vi "AlliGator Image Actions.vi"(0 "AlliGator Q Elements":T4[](array[typedef]), 1 "VI in":refnum<vi>, 2 "Script in":bool, 5 "AlliGator IV DVR in":refnum<data-value>, 7 "AlliGator Q Event in":T5=enum."GUI:Idle", 9 "Data":variant, 11 "error in (no error)":errorcluster, 12 "AlliGator Ctrl Refnums":T6) -> (3 "Script out":bool, 4 "Alligator Queue Elements":T4[](array[typedef]), 6 "AlliGator IV DVR out":refnum<data-value>, 10 "[Notebook Message]":T1[](array[typedef]) {"Message Style"."Text Alignment" items=["Left", "Right", "Center"]}, 15 "error out":errorcluster)   [LabVIEW 2021, in "AlliGator Action Engine.lvlib"]
doc: "Processes AlliGator source image-related actions."
uses:
  AlliGator Action Engine.lvlib
  AlliGator Internal Variables v2.ctl
  <vilib>/vision/Image Controls.llb/IMAQ Image.ctl
  AlliGator Gate Image Set.ctl
  AlliGator FLI Dataset Type.ctl
  AlliGator Data Series Type.ctl
  AlliGator Dataset Channel.ctl
  AlliGator Gate Arithmetic.ctl
  AlliGator Displayed Image.ctl
  Image/Named ROI Description.ctl
  AlliGator Decay Metadata v3.ctl
  AlliGator Decay Background Subtraction Info.ctl
  AlliGator Baseline Subtraction Method.ctl
  Graphs/XY Graph/XY Graph Plot Shift Parameters.ctl
  Graphs/XY Graph/XY Graph Plot Shift Method.ctl
  AlliGator Decay Extrapolation Parameters.ctl
  Phasor/Calibration Phasor (m, phi).ctl
  Phasor/Phasor Reference Series.ctl
  Phasor/Phasor Calibration Map v2.ctl
  Phasor/Phasor (g, s).ctl
  AlliGator Raw Phasor Plot Data v4.ctl
  Phasor/Phasor Standard Deviation Options.ctl
  AlliGator Phasor Multi-Harmonic Data.ctl
  Phasor/Phasor Harmonic Data.ctl
  AlliGator Decay Fit Options & Parameters v2.ctl
  Fits/IRF(X)PSED/Decay Fit Options v2.ctl
  Fits/Decay Convolution/Decay Model.ctl
  Fits/Residual Type.ctl
  Fits/IRF(X)PSED/Fit Weights Type.ctl
  Fits/Non-linear Fitting Method v2.ctl
  Fits/Fit Calculation Method.ctl
  Fits/Non-linear Fitting Algorithm.ctl
  AlliGator Decay Fit Parameter Constraints 2.ctl
  Fits/IRF(X)PSED/Decay Fit Parameters In List.ctl
  Fits/IRF(X)PSED/MLE Baseline Offset Type.ctl
  AlliGator Decay Preprocessing Parameters.ctl
  Fits/IRF(X)PSED/Decay Fit Parameters & Derived Quantities List.ctl
  AlliGator Parameter Maps Data.ctl
  AlliGator Q Event.ctl
  AlliGator Ctrl Refnums.ctl
  AlliGator Other Ctrl Refnums.ctl
  AlliGator State Indicator.ctl
  AlliGator Main Window Tabs.ctl
  AlliGator Phasor Plot Ctrl Refnums.ctl
  AlliGator Phasor Graph Ctrl Refnums.ctl
  Phasor/Phasor Calibration Type.ctl
  AlliGator Dataset Ctrl Refnums.ctl
  AlliGator Registered Events Ctrl Refnums.ctl
  AlliGator Image Histogram Control Refnums.ctl
  Histograms/Linear Histogram Options.ctl
  Histograms/Histogram Bin Option.ctl
  Histograms/Histogram Bin Position.ctl
  AlliGator Decay Fit Map Control Refnums.ctl
  AlliGator Q Element.ctl
  Notebook/Notebook Message Object.ctl
  Rich Text Box/Text Formatting.ctl
  Rich Text Box/Text Colors.ctl
  Alligator Elements Order in Action Stack.ctl
  AlliGator Variables List.ctl
  Palette/Image Palette Information.ctl
  Image/Image Display Palette Type.ctl
  Image/Image Display to Clipboard Options.ctl
  AlliGator Settings List.ctl
  AlliGator ROI Manager Actions.ctl
  Image/Image Control ROI Description.ctl
  Image/Image Save File Format.ctl
  AlliGator Saved TIFF Image Type.ctl
  AlliGator Selected ROI.ctl
  Image/Image Control Refnum.ctl
  Utilities/Read-Write.ctl
  5e39216f-2ed3-4ea3-88fe-69bdc2580e7f.vi
  Variant/Variant to Data/Variant to [String].vi
  Variant/Variant to Data/Variant to String.vi
  AlliGator Add Single Action to Stack.vi
  Variant/Variant to Data/Variant to Boolean.vi
  Variant/Variant to Data/Variant to DBL.vi
  AlliGator Source Image ROI Storage [SGL] v3.vi
  AlliGator Add Action Array to Stack.vi
  Variant/Variant to Data/Variant to I32.vi
  <vilib>/Utility/error.llb/Error Cluster From Error Code.vi
  <vilib>/ErrorRing/Error Ring.xnode
  Image/Image.lvlib
  Variant/Variant to Data/Variant to Data.lvlib
  GUI/GUI.lvlib
  AlliGator Files.lvlib
  AlliGator Image Profile Window.lvlib
  AlliGator Source Image.lvlib
  AlliGator Globals, Variables & Constants.lvlib
  Palette/Palette.lvlib
  AlliGator Settings.lvlib
  Rich Text Box/Rich Text Box.lvlib
  AlliGator ROIs.lvlib
  AlliGator Notebook.lvlib
  AlliGator Internal Variables.lvlib
  AlliGator Python Plugins.lvlib
  AlliGator Phasor Calibration.lvlib
  Utilities/Utilities.lvlib
  AlliGator GUI.lvlib
  Phasor/Phasor.lvlib
  AlliGator Decay Preprocessing.lvlib
  Graphs/XY Graph/XY Graph Add-Ons.lvlib
  AlliGator Phasor Graph.lvlib
  AlliGator Phasor Plot.lvlib
  Fits/Fits.lvlib
  AlliGator Decay Fit.lvlib
  AlliGator Decay Fit Parameter Map.lvlib
  AlliGator Dual-Channel Datasets.lvlib
  Histograms/Histogram Window.lvlib
  Notebook/Notebook.lvlib
panel:
  # "Drop the content of this VI on AlliGator's diagram\nIn AlliGator, replace the subVI template by a new version"
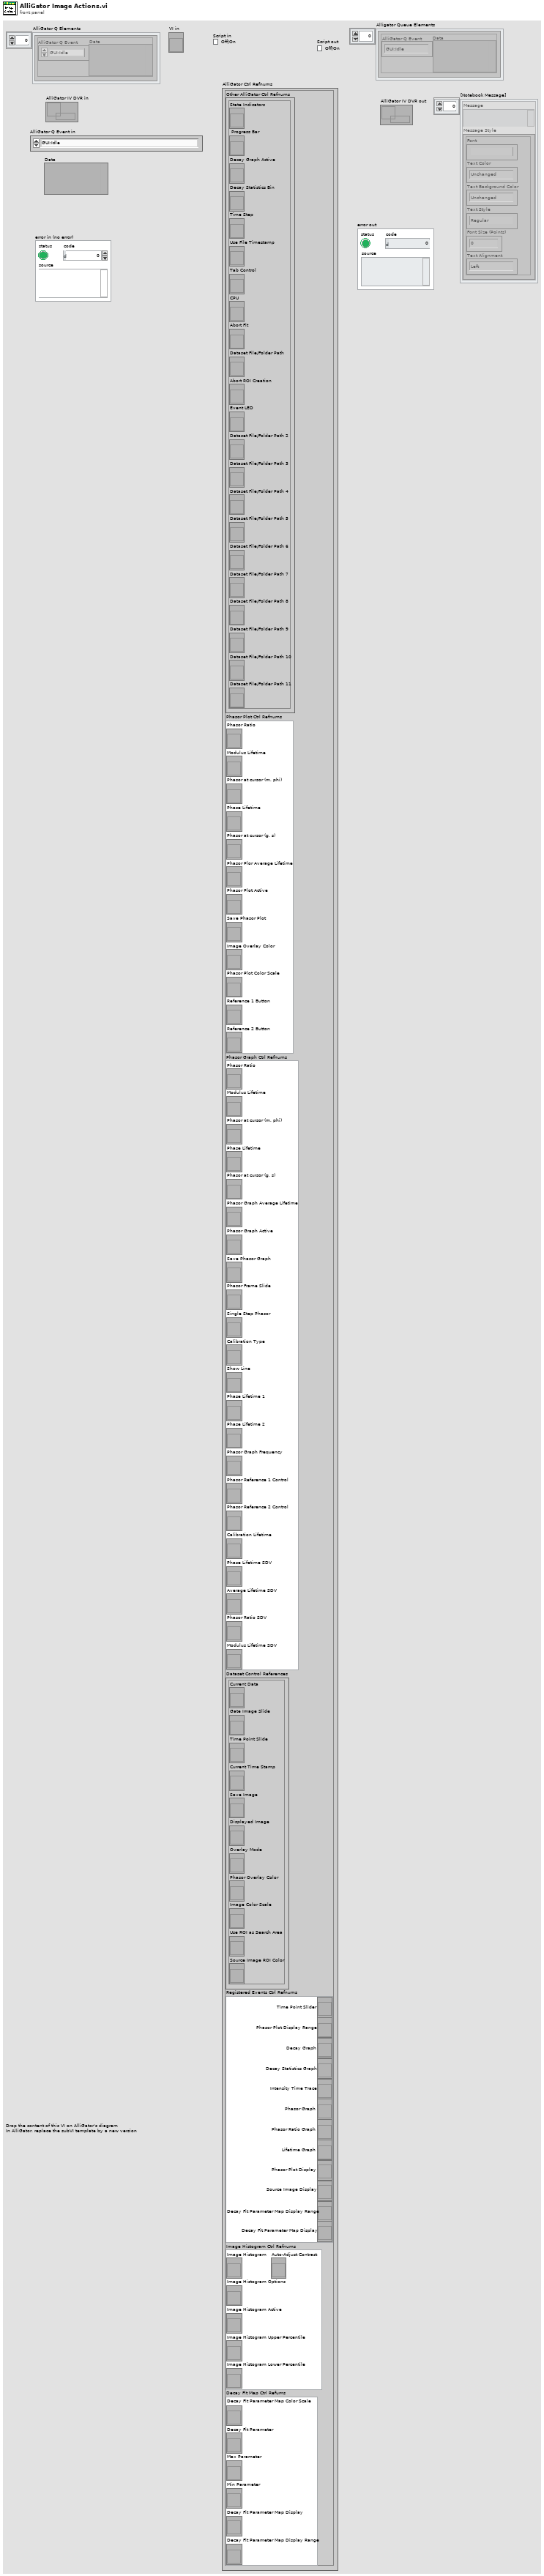
[diagram p1: front panel]
types:
  T1 = typedef "Notebook.lvlib/Notebook Message Object.ctl" = cluster{"Message":string, "Message Style":T2}
  T2 = typedef "Rich Text Box.lvlib/Text Formatting.ctl" = cluster{"Font":string, "Text Color":T3, "Text Background Color":T3, "Text Style":enum16{"Regular", "Bold", "Italic", "Underline", "Strikeout"}, "Font Size (Points)":dbl, "Text Alignment":i32}
  T3 = typedef "Rich Text Box.lvlib/Text Colors.ctl" = enum16{"Unchanged", "Black", "Blue", "Brown", "Gray", "Green", "Orange", "Pink", "Red", "White"}
  T4 = typedef "AlliGator Action Engine.lvlib/AlliGator Q Element.ctl" = cluster{"AlliGator Q Event":T5, "Data":variant}
  T5 = typedef "AlliGator Action Engine.lvlib/AlliGator Q Event.ctl" = enum16{"---- Files ----", "Files:Set Batch Export Files To Save", "Files:Set Dataset Loading & Pre-processing Options", "Files:Check #Frames in Dataset", "Files:Increment Frame Index", "Files:Open Mask Image", "Files:Open White Light Image", "Files:Open Single Dataset", "Files:New Folder of Folders Selected", "Files:Load File (all Types)_Scriptable", "Files:Move Flattened Series to Folders Series", "Files:Select Folder", "Files:Load FLI Dataset", "Files:Load Swiss SPAD 1 Dataset", "Files:Load Swiss SPAD 2 Dataset", "Files:Load .sdt FLI Dataset", "Files:Load .ptu FLI Dataset", "Files:Load .bin FLI Dataset", "Files:Load Single Gate Image Folder", "Files:Load I/m/phi Dataset (deprecated)", "Files:Load Single Image", "Files:Subtract Background File", "Files:Export FLI Dataset", "Files:Load HDF5 FLI Dataset", "Files:Set Destination File Path", "Files:Save Mask Image", "Files:Batch Conversion", "Files:New Folder Selected", "Files:Close FLI Dataset", "Files:Close FLI Dataset Series", "Files:Close White Light Image", "Files:Close Mask Image", "---- FLI Dataset ----", "FLI Dataset:Channel Arithmetic", "FLI Dataset:Export Average Lifetime Map as ASCII", "FLI Dataset:Export User-Defined Quantity Map as ASCII", "FLI Dataset:Python Function FLI Dataset Event", "FLI Dataset:ROI Analysis", "FLI Dataset:Tilted Logistic Square Gated IRF Characteristics Map", "FLI Dataset:Logistic Square Gated IRF Characteristics Map", "FLI Dataset:Square Gated IRF Characteristics Map", "FLI Dataset:Multi-ROI Single-Pixel Phasor Analysis", "FLI Dataset:Multi-ROI Single-Pixel NLSF Analysis", "FLI Dataset:All ROIs IRF Extraction", "FLI Dataset:All ROIs Decay Fit Non-Interactive (Fast + Individual IRF)", "FLI Dataset:All ROIs Phasor Analysis", "FLI Dataset:All ROIs Decay Fit", "FLI Dataset:Fluorescence Decay Statistics", "FLI Dataset:Update Decay Statistics Graph", "FLI Dataset:Get Decay from ROI", "FLI Dataset:All ROIs Average Lifetimes", "---- FLI Dataset Series ----", "FLI Dataset Series:Sum All Datasets in Series", "FLI Dataset Series:Add Dataset to Accumulated Dataset", "FLI Dataset Series:Display Accumulated Dataset", "FLI Dataset Series:Clear Dataset Series Sum", "FLI Dataset Series:Time-Series Analysis (NLSF)", "FLI Dataset Series:Time-Series Analysis (Phasor)", "---- Image ----", "Image:Update Image Profile Plots", "Image:Image Histogram Cursor Move", "Image:Image Histogram", "Image:Image Contrast", "Image:Set Image Histogram Cursor Move Flag", "Image:Clear Image Overlay", "Image:Use ROI as Search Area", "Image:Set ROI Diameter", "Image:Save Image Data as TIFF", "Image:Save Displayed Image with Overlay", "Image:Save Image Overlay Only", "Image:Save Image as Hot Pixel Mask", "Image:Change Source Image Color Palette", "Image:Copy Image to Clipboard", "Image:Source Image ROI Selection", "Image:Delete All ROIs", "Image:Delete All Unselected ROIs", "Image:Delete ROI", "Image:Merge All ROIs", "Image:Store ROI", "Image:Source Image ROI Storage", "Image:Export ROI Description to Notebook", "Image:Save ROI", "Image:Load ROI", "Image:Paste ROI Definition", "Image:Clear ROI", "Image:Identify ROIs in Mask Image", "Image:Create Complementary ROI", "Image:Create Contour ROI", "Image:Create ROI(s) from Pixels with Peak above Min_Scriptable", "Image:Create ROI(s) from Pixels with Intensity above Min_Scriptable", "Image:Compute ROI Statistics", "Image:Delete ROI(s) based on ROI Characteristics", "Image:Create ROI Grid", "Image:ROI to Individual Pixel ROIs", "Image:Python Function Source Image Event", "Image:Show Phasor Calibration Map ROI Centers", "Image:Convert ROI to Mask Image", "Image:Mouse Move", "Image:Mouse Up", "Image:Set Source Image Mouse Move Flag", "Image:Add Scale Bar Overlay", "Image:Delete Existing ROIs Option", "Image:Overlay ROI Median", "---- Decay ----", "Decay:Clear IRF/Reference Plot", "Decay:Clear Local IRFs", "Decay:Add Decay to Graph", "Decay:Smoothen Plot", "Decay:Smoothen Plot Tail", "Decay:Average Selected Plots", "Decay:Extract IRF", "Decay:Optimal IRF Extraction", "Decay:Threshold IRF", "Decay:Fit to Model IRF", "Decay:Fit IRF to Square Gate", "Decay:Fit IRF to Logistic Square Gate", "Decay:Fit IRF to Tilted Logistic Square Gate", "Decay:Create Bounding Cursors Set", "Decay:Export Bounding Cursors Definition to Notebook", "Decay:Denoise Plot", "Decay:Compute Cumulative Function", "Decay:Use as Reference Decay", "Decay:Show Reference Decay/IRF", "Decay:Extrapolate Decay", "Decay:Create Head & Tail Bounding Cursors", "Decay:Store Cursor-defined Head & Tail Fractions", "Decay:Rebin Plot", "Decay:1-Normalize Decay", "Decay:[0-1]-Normalize Plot", "Decay:Straighten Decay", "Decay:Shift Decay", "Decay:Fold Decay", "Decay:Fit Decay", "Decay:Global Fit of Selected Decays", "Decay:Post Global Fit Script", "Decay:Add Global Fit Parameters to Graph", "Decay:Add Decay Parameter(s) to Plot (Graph)", "Decay:Export Decay to Phasor Graph", "Decay:Plot Decay Shifts", "Decay:Compute Average Lifetime", "Decay:Plot Convolution", "Decay:Graph Tip Strip Update", "---- Decay Statistics ----", "Decay Statistics:Tip Strip Update", "---- Intensity Time Trace ----", "Intensity Time Trace:Use File Timestamp", "Intensity Time Trace:Load Intensity Corrections File", "Intensity Time Trace:Clear Intensity Corrections File", "Intensity Time Trace:Tip Strip Update", "---- Phasor Plot ----", "Phasor Plot:Build Phasor Plot", "Phasor Plot:Change Phasor Plot Color Palette", "Phasor Plot:Adjust Phasor Plot Display Range", "Phasor Plot:Highlight Image ROI in Phasor Plot", "Phasor Plot:Save Phasor Plot Image with Overlay", "Phasor Plot:Export Complex Phasor Map", "Phasor Plot:Export Phasor Ratio Map", "Phasor Plot:Export Average Lifetime Map", "Phasor Plot:Compute Phase Lifetime Histogram", "Phasor Plot:Compute Phasor Ratio Histogram", "Phasor Plot:Compute Phase Lifetime vs Intensity Scatter Plot", "Phasor Plot:Weber 2-Component Decomposition", "Phasor Plot:Update Phasor Color Map Vertices", "Phasor Plot:Clear Phasor Overlay", "Phasor Plot:Use Segment Extremities as References", "Phasor Plot:Use UC/Segment Intersections as References", "Phasor Plot:Use UC/Principal Axis Intersections as References", "Phasor Plot:Use UC/Linear Fit Intersections as References", "Phasor Plot:Update Phasor Plot Reference", "Phasor Plot:Show Local Phasor Info in Phasor Plot", "Phasor Plot:Update Phasor Plot State", "Phasor Plot:Phasor Plot ROI Storage", "Phasor Plot:Phasor Plot ROI Selection", "Phasor Plot:Python Function Phasor Plot Event", "Phasor Plot:Overlay Phasor ROI, Ratio or Map in Source Image", "Phasor Plot:Compute Decay of Selected Phasors", "Phasor Plot:Phasor at Image Pixel", "Phasor Plot:Mouse Move", "Phasor Plot:Mouse Up", "Phasor Plot:Display Range Mouse Move", "Phasor Plot:Set Mouse Move Flag", "---- Phasor Graph ----", "Phasor Graph:Calibrated Phasor Map Series", "Phasor Graph:Whole Image Phasor Scatter Plot (Todo)", "Phasor Graph:Get Phasor Value", "Phasor Graph:Create New Phasor Plot Dialog", "Phasor Graph:Update Last Phasor Value", "Phasor Graph:Update Phasor (m, phi)", "Phasor Graph:Remove Single Phasor from Plot", "Phasor Graph:Add Single Phasor to Plot", "Phasor Graph:Remove Phasor Plot", "Phasor Graph:Remove Selected Phasor Plots", "Phasor Graph:Clear Phasor Data", "Phasor Graph:Clear Phasor Graph", "Phasor Graph:Cursor Move", "Phasor Graph:Draw Cursor Connecting Line", "Phasor Graph:Clear Cursor Connecting Line", "Phasor Graph:Find UC Intersection", "Phasor Graph:Use UC/Cursor-Defined Line Intersections", "Phasor Graph:Use Selected Plots Fitted Line/UC Intersections", "Phasor Graph:Use Selected Plots Principal Axis/UC Intersections", "Phasor Graph:Show Single Phasor", "Phasor Graph:Save Single Phasor Plot", "Phasor Graph:Save All Phasor Plots", "Phasor Graph:Load Phasor Plot(s)", "Phasor Graph:Phasor Multiplication", "Phasor Graph:Compute Average Phasor", "Phasor Graph:Compute Multiple Average Phasors (Selected Plots)", "Phasor Graph:Export Single Phasor Plot Phase Lifetimes", "Phasor Graph:Phase Lifetime Trajectory", "Phasor Graph:Phase Lifetime vs Intensity Scatter Plot (deprecated)", "Phasor Graph:Parameter 2 vs Parameter 1 Scatter Plot", "Phasor Graph:Use Cursor n Location", "Phasor Graph:Set Reference n to Current Phase Lifetime Value", "Phasor Graph:Set Reference n to Lifetime Value", "Phasor Graph:Set Cursor n Location", "Phasor Graph:Save Phasor Graph Image", "Phasor Graph:Update SEPL Plot", "Phasor Graph:Export Single Phasor Plot Data", "Phasor Graph:Export Selected Phasor Plots Data", "Phasor Graph:Python Function Phasor Graph Event", "Phasor Graph:Tip Strip Update", "---- Calibration ----", "Calibration:Set Calibration Type", "Calibration:Load/Save Phasor Calibration", "Calibration:Load/Save Phasor Calibration Series", "Calibration:Load/Save Phasor Calibration Map", "Calibration:Use as Calibration", "Calibration:Compute Optimal Calibration from Phasor References", "Calibration:Clear Phasor Calibration", "Calibration:Single Phasor Calibration Information", "Calibration:Use as Calibration Series", "Calibration:Use as Calibration Map", "Calibration:Clear Calibration Series", "Calibration:Phasor Calibration Series Information", "Calibration:Clear Calibration Map", "Calibration:Phasor Calibration Map Information", "Calibration:Apply Phasor Calibration", "Calibration:Update Single Plot Calibration", "Calibration:Update Multiple Plots Calibration", "Calibration:Clear Single Plot Calibration", "Calibration:Clear All Plots Calibrations", "Calibration:Clear Plot(s) Calibration(s)?", "Calibration:Phasor Calibration Maps (# Gates Series)", "---- Phasor Ratio ----", "Phasor Ratio:Clear Reference n", "Phasor Ratio:Toggle Selected Plot(s)  Lock to Reference 1", "Phasor Ratio:Use as Reference n", "Phasor Ratio:Send Reference n to Notebook", "Phasor Ratio:Toggle Selected Plot(s)  Lock to Reference 2", "Phasor Ratio:Compute Phasor Ratio at Mouse Location", "Phasor Ratio:Compute Phasor Plot's Average Phasor Ratio", "Phasor Ratio:Compute Time-Series Phasor Ratios", "Phasor Ratio:Fit Line to Phasor Ratio Plot", "Phasor Ratio:Save References", "Phasor Ratio:Load References", "Phasor Ratio:Update Phasor Reference 1", "Phasor Ratio:Update Phasor Reference 2", "Phasor Ratio:Move Cursor n to Reference n", "Phasor Ratio:Use as Phasor Reference 1 Lifetime", "Phasor Ratio:Use as Phasor Reference 2 Lifetime", "Phasor Ratio:Export Phasor Ratio Map as ASCII", "Phasor Ratio:Tip Strip Update", "---- Lifetime & Other Parameters Graph ----", "Lifetime:Tip Strip Update", "---- Decay Fit Parameter Map ----", "Decay Fit Parameter Map:Export ROI NLSF Data as ASCII", "Decay Fit Parameter Map:Set Decay Fit  Parameter Map Selection", "Decay Fit Parameter Map:Build Decay Fit Parameter Map", "Decay Fit Parameter Map:Change Decay Fit Parameter Map Color Palette", "Decay Fit Parameter Map:Export Decay Fit Parameter Map Data as ASCII", "Decay Fit Parameter Map:Export All Decay Fit Parameter Maps Data as ASCII", "Decay Fit Parameter Map:Send Map Data to Lifetime Graph", "Decay Fit Parameter Map:Save Decay Fit Parameter Map Image", "Decay Fit Parameter Map:Save-Load IRFs & Fit Data", "Decay Fit Parameter Map:Update Local Decay Plots", "Decay Fit Parameter Map:Python Function Decay Fit Parameters Map Event", "Decay Fit Parameter Map:Overlay Decay Fit Parameter Map in Source Image", "Decay Fit Parameter Map:Plot Map Data vs Intensity", "Decay Fit Parameter Map:Mouse Up", "Decay Fit Parameter Map:Display Range Mouse Move", "---- Generic Graph ----", "Generic Graph:Generic XY Graph Event", "Generic Graph:Python Function XY Graph Event", "Generic Graph:New Plot", "Generic Graph:Save Plot", "Generic Graph:XY Plot Histogram", "Generic Graph:Set XY Graph Plot Name", "Generic Graph:Set Last Cursor Style", "Generic Graph:Tip Strip Update", "---- GUI ----", "GUI:Start Script", "GUI:Type of Displayed Image Changed", "GUI:Gate Image Slide Changed", "GUI:Show Busy Icon", "GUI:Show Busy Icon & Abort Button", "GUI:Hide Busy Icon", "GUI:Hide Busy Icon & Abort Button", "GUI:Abort", "GUI:End Script", "GUI:Start Timing", "GUI:End Timing", "GUI:Set State Indicator", "GUI:Send Parameters JSON Strings to Clipboard", "GUI:Set Gate Step", "GUI:Idle", "GUI:Initialization", "GUI:Quit", "GUI:Increment Dataset Index", "GUI:Set Dataset Index to -1", "GUI:Time Series Slider Moved", "GUI:Time Series Slider Changed", "GUI:Toggle Playback or Loop", "GUI:Playback Script", "GUI:Set Phasor Frequency", "GUI:Open Window", "GUI:Start Test Script", "GUI:End Test Script", "DEBUG"}
  T6 = typedef "AlliGator GUI.lvlib/AlliGator Ctrl Refnums.ctl" = cluster{"Other AlliGator Ctrl Refnums":T7, "Phasor Plot Ctrl Refnums":T8, "Phasor Graph Ctrl Refnums":T9, "Dataset Control References":T10, "Registered Events Ctrl Refnums":T11, "Image Histogram Ctrl Refnums":T12, "Decay Fit Map Ctrl Refums":T13}
  T7 = typedef "AlliGator GUI.lvlib/AlliGator Other Ctrl Refnums.ctl" = cluster{"State Indicators":refnum<vi>, " Progress Bar":refnum<vi>, "Decay Graph Active":refnum<vi>, "Decay Statistics Bin":refnum<vi>, "Time Step":refnum<vi>, "Use File Timestamp":refnum<vi>, "Tab Control":refnum<vi>, "CPU":refnum<vi>, "Abort Fit":refnum<vi>, "Dataset File/Folder Path":refnum<vi>, "Abort ROI Creation":refnum<vi>, "Event LED":refnum<vi>, "Dataset File/Folder Path 2":refnum<vi>, "Dataset File/Folder Path 3":refnum<vi>, "Dataset File/Folder Path 4":refnum<vi>, "Dataset File/Folder Path 5":refnum<vi>, "Dataset File/Folder Path 6":refnum<vi>, "Dataset File/Folder Path 7":refnum<vi>, "Dataset File/Folder Path 8":refnum<vi>, "Dataset File/Folder Path 9":refnum<vi>, "Dataset File/Folder Path 10":refnum<vi>, "Dataset File/Folder Path 11":refnum<vi>}
  T8 = typedef "AlliGator GUI.lvlib/AlliGator Phasor Plot Ctrl Refnums.ctl" = cluster{"Phasor Ratio":refnum<vi>, "Modulus Lifetime":refnum<vi>, "Phasor at cursor (m, phi)":refnum<vi>, "Phase Lifetime":refnum<vi>, "Phasor at cursor (g, s)":refnum<vi>, "Phasor Plor Average Lifetime":refnum<vi>, "Phasor Plot Active":refnum<vi>, "Save Phasor Plot":refnum<vi>, "Image Overlay Color":refnum<vi>, "Phasor Plot Color Scale":refnum<vi>, "Reference 1 Button":refnum<vi>, "Reference 2 Button":refnum<vi>}
  T9 = typedef "AlliGator GUI.lvlib/AlliGator Phasor Graph Ctrl Refnums.ctl" = cluster{"Phasor Ratio":refnum<vi>, "Modulus Lifetime":refnum<vi>, "Phasor at cursor (m, phi)":refnum<vi>, "Phase Lifetime":refnum<vi>, "Phasor at cursor (g, s)":refnum<vi>, "Phasor Graph Average Lifetime":refnum<vi>, "Phasor Graph Active":refnum<vi>, "Save Phasor Graph":refnum<vi>, "Phasor Frame Slide":refnum<vi>, "Single Step Phasor":refnum<vi>, "Calibration Type":refnum<vi>, "Show Line":refnum<vi>, "Phase Lifetime 1":refnum<vi>, "Phase Lifetime 2":refnum<vi>, "Phasor Graph Frequency":refnum<vi>, "Phasor Reference 1 Control":refnum<vi>, "Phasor Reference 2 Control":refnum<vi>, "Calibration Lifetime":refnum<vi>, "Phase Lifetime SDV":refnum<vi>, "Average Lifetime SDV":refnum<vi>, "Phasor Ratio SDV":refnum<vi>, "Modulus Lifetime SDV":refnum<vi>}
  T10 = typedef "AlliGator GUI.lvlib/AlliGator Dataset Ctrl Refnums.ctl" = cluster{"Current Data":refnum<vi>, "Gate Image Slide":refnum<vi>, "Time Point Slide":refnum<vi>, "Current Time Stamp":refnum<vi>, "Save Image":refnum<vi>, "Displayed Image":refnum<vi>, "Overlay Mode":refnum<vi>, "Phasor Overlay Color":refnum<vi>, "Image Color Scale":refnum<vi>, "Use ROI as Search Area":refnum<vi>, "Source Image ROI Color":refnum<vi>}
  T11 = typedef "AlliGator GUI.lvlib/AlliGator Registered Events Ctrl Refnums.ctl" = cluster{"Time Point Slider":refnum<vi>, "Phasor Plot Display Range":refnum<vi>, "Decay Graph":refnum<vi>, "Decay Statistics Graph":refnum<vi>, "Intensity Time Trace":refnum<vi>, "Phasor Graph":refnum<vi>, "Phasor Ratio Graph":refnum<vi>, "Lifetime Graph":refnum<vi>, "Phasor Plot Display":refnum<vi>, "Source Image Display":refnum<vi>, "Decay Fit Parameter Map Display Range":refnum<vi>, "Decay Fit Parameter Map Display":refnum<vi>}
  T12 = typedef "AlliGator GUI.lvlib/AlliGator Image Histogram Control Refnums.ctl" = cluster{"Image Histogram":refnum<vi>, "Image Histogram Options":refnum<vi>, "Image Histogram Active":refnum<vi>, "Image Histogram Upper Percentile":refnum<vi>, "Image Histogram Lower Percentile":refnum<vi>, "Auto-Adjust Contrast":refnum<vi>}
  T13 = typedef "AlliGator Decay Fit Parameter Map.lvlib/AlliGator Decay Fit Map Control Refnums.ctl" = cluster{"Decay Fit Parameter Map Color Scale":refnum<vi>, "Decay Fit Parameter":refnum<vi>, "Max Parameter":refnum<vi>, "Min Parameter":refnum<vi>, "Decay Fit Parameter Map Display":refnum<vi>, "Decay Fit Parameter Map Display Range":refnum<vi>}
  T14 = typedef "AlliGator Action Engine.lvlib/Alligator Elements Order in Action Stack.ctl" = enum16{"Enqueue 2 AFTER 1", "Enqueue 2 BEFORE 1"}
  T15 = typedef "AlliGator Globals, Variables & Constants.lvlib/AlliGator Variables List.ctl" = enum16{"---- GUI ----", "GUI:Initialization Status", "GUI:State Indicators Refnum", "GUI:Original AlliGator Menu Items", "GUI:Current Action Loop State", "GUI:Script in progress", "GUI:Playback", "GUI:Loop Playback", "GUI:Search ROI Used", "GUI:Search ROI", "Decay Graph Max Legend Size", "Intensity Graph Max Legend Size", "Decay Statistics Graph Max Legend Size", "Phasor Graph Max Legend Size", "Phasor Ratio Graph Max Legend Size", "Lifetime Graph Max Legend Size", "---- Files ----", "Files:Export Dataset Frames as Individual Files", "Files:Show Batch Export Help Balloons", "Files:Frames in Dataset", "Files:ptu File Frame Start Indices", "Files:Current Frame in Dataset", "Files:Current Frame Timestamp", "Files:Dataset Loaded", "Files:Dataset Metadata", "Files:Dataset Channel", "Files:Dataset Data Description", "Files:Background Dataset Metadata", "Files:Background Dataset Channel", "Files:Background Dataset Data Description", "Files:Background File Subtraction", "Files:Background File Path", "Files:Background File Pile-up Correction", "Files:Background File Pixel Well Capacity", "Files:Background File Scaling Factor", "Files:Current Dataset Load Settings", "Files:Dataset Path", "Files:ICCD-specific Information", "Files:Macrotime Gate Separation", "------ Python Plugins ------", "Python Plugins:Information", "Python Plugins:Python Session", "Python Plugins:Valid Python Session?", "---- Source Image ----", "Source Image:ROIs", "Source Image:Current ROI", "Source Image:ROI Event Refnum", "X_Source Image Display Range", "X_Source Image Palette Information", "X_Type of Displayed Image", "X_Time Gate Slider", "Source Image:Palette List", "Source Image:Scale", "Source Image:ROI Overlay Color", "Source Image:Overlay to Erase", "Source Image:Is Displayed Image Accumulated", "Source Image:White Light Image Modified", "Source Image:Mask Image Modified", "---- Image Profile Window ----", "Image Profile:Window Event Refnum", "Image Profile:IntensityType", "Image Profile:Intensity Average Type", "Image Profile:Intensity-weighted SDV", "Image Profile:Box Profile Type", "Image Profile:Window Open", "Image Profile:Plotted Fit Parameter", "------ Phasor Graph -------", "Phasor Graph:Show Line", "---- Phasor Plot ---", "Phasor Plot:Parameters Changed", "Phasor Plot:FLI Dataset Modified since last Calculation", "Phasor Harmonics Data", "Selected Phasor Harmonics", "Phasor Harmonic Manager Event Refnum", "Phasor Plot:ROIs", "Phasor Plot:Current ROI", "Phasor Plot:ROI Event Refnum", "Phasor Plot:Image Reference Points", "Phasor Plot:Computed", "Phasor Plot:Palette Information", "Phasor Plot:Palette List", "Phasor Plot:Phasor Ratio Palette Information", "Phasor Plot:Phasor Ratio Palette List", "Phasor Plot:Image Scale", "Phasor Plot:Image Overlay to Erase", "Phasor Plot:Image Elements to Update", "Phasor Plot:Current Calculation Parameters", "Phasor Plot:Current Calibration Options", "Phasor Plot:Reset Cumulated Phasor Plot", "Phasor Plot:Reference 1", "Phasor Plot:Lifetime Reference 1", "Phasor Plot:Reference 1 Frequency", "Phasor Plot:Reference 2", "Phasor Plot:Lifetime Reference 2", "Phasor Plot:Reference 2 Frequency", "---- Decay Analysis ----", "Number of Selected Decays to Fit", "LS Fit Results", "LAR Fit Results", "BS Fit Results", "Last Decay Max - Min", "Best Fit Parameters", "Best Fit Parameter Names", "Actual Size X", "Actual Size Y", "Binning X", "Binning Y", "Actual # Gates", "Dataset Number", "Gates to...", "Gates Skipped", "Gates to keep", "Gate Step", "Gate Separation", "Reversed Gates", "Pile-up Correction", "Pixel Well Capacity", "Background Subtracted", "Background Subtraction Method", "Background Definition Range", "Background File (deprecated)", "Number of Dataset Accumulated", "Array of Accumulated Dataset Paths", "Do Averaged Datasets", "Destination File Path", "Process Plot Target", "Use 1/D as Phasor Frequency", "---- Decay Fit Parameter Map -----", "Decay Fit Parameter Map:Palette Information", "Decay Fit Parameter Map:Palette List", "------- Local Decay Window ---------", "Local Decay Graph Window:Event Refnum", "Local Decay Graph Window:Use normalized IRF for convolution", "----- Miscellaneous ----", "Misc:Skippable Dialog Windows Status"}
  T16 = typedef "Palette.lvlib/Image Palette Information.ctl" = cluster{"Palette Name [# Colors,int?,inv?]":string, "Palette Type":T17, "Palette Colors":u32[], "Interpolate?":bool}
  T17 = typedef "Image.lvlib/Image Display Palette Type.ctl" = u32
  T18 = typedef "Image.lvlib/Image Display to Clipboard Options.ctl" = cluster{"Include Overlay (T)":bool, "Image Only (T)":bool}
  T19 = cluster{"CtlRef":refnum<vi>, "Image to Clipboard Options":T18}
  T20 = typedef "AlliGator Settings.lvlib/AlliGator Settings List.ctl" = enum16{"GUI:Visible Settings Tab", "GUI:Last Run Version", "Source Image:Use Image Histogram for Contrast", "Source Image:Low Count Pixels Rejection Options", "Source Image:High Count Pixels Rejection Options", "Source Image:Use Image Brightness", "Source Image:Blend Overlay with Image Background", "Source Image:Use Fixed ROI Diameter", "Source Image:ROI Diameter", "Source Image:ROI Center Color", "Source Image:Peak Threshold", "Source Image:Intensity Threshold", "Source Image:Image Binning Options", "Source Image:Image Smoothing Options", "Source Image:Image Histogram Active", "Source Image:Invert Binary Mask", "Source Image:Hot Pixel Removal", "Source Image:Overlay Analyzed ROI Center", "Source Image:Auto-Adjust Contrast", "Source Image:Histogram Lower Percentile", "Source Image:Histogram Upper Percentile", "Source Image:Save Source Image", "Source Image:Scale Bar Options", "Source Image:Image Resolution (Pixel Size)", "Source Image:Flatfield Correction", "Source Image:Show Dead Left Columns Correction", "Source Image:Dead Left Columns Correction", "Source Image:Image Pre-Processing Operations Order", "Source Image:Overlay ROI Median", "Source Image:Median Overlay Color", "Data Information:Gate Width", "Data Information:Nanotime Gate Separation", "Data Information:Macrotime Gate Separation", "Data Information:Gate Step", "Data Information:# Gates", "Data Information:Gate Image Exposure", "Data Information:Gate Image Integration", "Data Information:Gates to Skip", "Data Information:Gates to Keep", "Data Information:Define Gates to", "Data Information:Channel Name", "Data Information:Available Channel Names", "Data Information:Channel Arithmetic", "Data Information:Background File Subtraction", "Data Information:Background File", "Data Information:Background Scaling Factor", "Data Information:Background Pile-up Correction", "Data Information:Background Pixel Well Capacity", "Data Information:Laser Period", "Data Information:SYNC Period", "Data Information:Pile-up Correction", "Data Information:Pixel Well Capacity", "Data Information:Dataset Scaling Factor", "Fluorescence Decay_Decay Pre-Processing:Reverse Gates", "Fluorescence Decay_Decay Pre-Processing:Verbose Decay Pre-Processing", "Fluorescence Decay_Decay Pre-Processing:Use Decay Pre-Processing", "Fluorescence Decay_Decay Pre-Processing:Background Subtraction", "Fluorescence Decay_Decay Pre-Processing:Background Definition Range", "Fluorescence Decay_Decay Pre-Processing:Baseline Subtraction Method", "Fluorescence Decay_Decay Pre-Processing:Decay Pre-Processing Operations Order", "Fluorescence Decay_Decay Pre-Processing:Smoothing Parameter", "Fluorescence Decay_Decay Pre-Processing:Shift Decay", "Fluorescence Decay_Decay Pre-Processing:Decay Shift Parameters", "Fluorescence Decay_Decay Pre-Processing:Fold Decay", "Fluorescence Decay_Decay Pre-Processing:# Folds", "Fluorescence Decay_Decay Pre-Processing:1-Normalize Decay", "Fluorescence Decay_Decay Pre-Processing:[0-1]-Normalize Decay", "Fluorescence Decay_Decay Pre-Processing:Smoothen Decay", "Fluorescence Decay_Decay Pre-Processing:Extrapolate Decay", "Fluorescence Decay_Decay Pre-Processing:Use Periodicity", "Fluorescence Decay_Decay Pre-Processing:Use Cursors", "Fluorescence Decay_Decay Pre-Processing:Tail Fraction", "Fluorescence Decay_Decay Pre-Processing:Head Fraction", "Fluorescence Decay_Decay Pre-Processing:Additional Points", "Fluorescence Decay_Decay Pre-Processing:Straighten Decay", "Fluorescence Decay_Decay Pre-Processing:Constant Background", "Fluorescence Decay_Decay Pre-Processing:Pixel-Normalize Decay", "Fluorescence Decay_Advanced Analysis:Extract IRF instead of Decay", "Fluorescence Decay_Advanced Analysis:IRF Extraction Options", "Fluorescence Decay_Advanced Analysis:IRF Optimization Options", "Fluorescence Decay_Advanced Analysis:Square Pulse Options", "Fluorescence Decay_Advanced Analysis:IRF Order", "Fluorescence Decay_Advanced Analysis:IRF Time Constants", "Fluorescence Decay_Advanced Analysis:Wavelet Analysis Options", "Fluorescence Decay_Advanced Analysis:Average Lifetime Options", "Fluorescence Decay_Fit Options:Fit Options", "Fluorescence Decay_Fit Options:Use Legacy Fitting Approach", "Fluorescence Decay_Fit Options:Use Data Information Laser Period", "Fluorescence Decay_Fit Parameters:Displayed Fit Parameters", "Fluorescence Decay_Fit Parameters:Fit Parameter Constraints", "Fluorescence Decay_Fit Parameters:Export Tabulated Results", "Fluorescence Decay_Fit Parameters:MLE Baseline Offset Type", "Fluorescence Decay_Fit Parameters:MLE Baseline Offset", "Fluorescence Decay_Fit Parameters:Guess Parameter Names", "Fluorescence Decay_Fit Parameters:Guess Parameter Values", "Fluorescence Decay_Fit Parameters:Guess Parameters Options", "Fluorescence Decay_Styles:Show Last Decay Only", "Fluorescence Decay_Styles:Decay Graph Color Array", "Fluorescence Decay:Decay Graph Active", "Fluorescence Decay Statistics:Min Peak Value", "Fluorescence Decay Statistics:Reject Low Decay Peak Pixels", "Fluorescence Decay Statistics:Reject High Decay Peak Pixels", "Fluorescence Decay Statistics:Max Peak Value", "Time Traces:Use File Timestamp", "Time Traces:Time Step", "Time Traces:Use Intensity Correction File", "Time Traces:Intensity Correction File", "Phasor Plot:Phasor Plot Smoothing Options", "Phasor Plot:Phasor Plot Size", "Phasor Plot:Phasor Plot Graphics Options", "Phasor Plot:Cumulative Phasor Plot", "Phasor Plot:Use Phasor Brightness", "Phasor Plot:Blend Overlay with Phasor Background", "Phasor Plot:Save Phasor Plot", "Phasor Plot:Show References", "Phasor Plot:Phasor Ratio Decay Range", "Phasor Plot:Exponential Fading", "Phasor Plot:Phasor Ratio Reference Colors", "Phasor Plot:Reference Radius", "Phasor Plot:Show Color Map Vertices", "Phasor Plot:Phasor Plot Active", "Phasor Plot:Phasor Ratio Color Map Type", "Phasor Plot:Phasor Ratio Color Map", "Phasor Plot:Phasor Ratio Display Range", "Phasor Plot:Selected Image ROI(s)", "Phasor Plot:All Image ROIs", "Phasor Plot:Selected Phasor Plot ROI(s)", "Phasor Plot:All Phasor Plot ROIs", "Phasor Plot:Phasor Ratio Color-Coded Quantity", "Phasor Plot:Store Phasor Harmonics", "Phasor Plot:Draw Reference Segment", "Phasor Plot:User-Defined Quantity", "Phasor Graph:Phasor Frequency", "Phasor Graph:Phasor Ratio Type", "Phasor Graph:Pixel-level Phasor Computation", "Phasor Graph:Save Phasor Graph", "Phasor Graph:Phasor Graph Active", "Phasor Graph:Phasor SDV Options", "Phasor Calibration:Use Backup Calibration if needed", "Phasor Graph:Define Shortest Lifetime as", "Phasor Calibration:Backup Calibration Type", "Phasor Calibration:Calibration Type", "Phasor Calibration:Calibration Lifetime", "Phasor Calibration:Calibration Map Algorithm", "Single-Exponential Phasor Locus (SEPL):Gate Parameters", "Single-Exponential Phasor Locus (SEPL):User-defined Gate", "Single-Exponential Phasor Locus (SEPL):User-defined IRF", "Single-Exponential Phasor Locus (SEPL):Phasor Parameters", "Single-Exponential Phasor Locus (SEPL):Decay & IRF Parameters", "Single-Exponential Phasor Locus (SEPL):Display Parameters", "Lifetime Analysis:Decay Analysis Parameters", "Lifetime Analysis:Lifetime Map Active", "Plugins:Python Settings", "Miscellaneous:Verbose Mode", "Miscellaneous:Beep after Script", "Miscellaneous:Saved Image File Format", "Miscellaneous:Exported Gate Image Settings", "Miscellaneous:Include Loading in Timing", "Miscellaneous:Verbose Settings Mode", "Miscellaneous:Histogram Options", "Miscellaneous:Beep on Error", "Miscellaneous:# Logical Processors Used", "Miscellaneous:ROI Description Max Characters", "Miscellaneous:Verbose Error Mode", "Miscellaneous:Transparent Mask Color"}
  T21 = typedef "AlliGator ROIs.lvlib/AlliGator ROI Manager Actions.ctl" = enum16{"Undefined", "Delete Current ROI", "Delete All Unselected ROIs", "Delete Multiple ROIs", "Delete All ROIs", "Swap ROIs", "Insert ROI", "Update Current ROI Descriptor", "Rename Current ROI", "Store New ROI", "Store Multiple ROIs", "Select Next ROI", "Select Previous ROI", "Find Selected ROI", "Show All ROIs", "Update ROI Manager Window", "Merge All ROIs", "Unmerge ROI", "Set Selected ROI by ID"}
  T22 = typedef "ROI Descriptor" = cluster{"Global Rectangle":i32[], "Contours":cluster{"ID":enum32{"External", "Internal"}, "Type":u32, "Coordinates":i32[]}[]}
  T23 = typedef "Image.lvlib/Image Control ROI Description.ctl" = cluster{"Image Control Label":string, "ROI Descriptor":T22}
  T24 = typedef "IMAQ Image.ctl" = refnum<image>
  T25 = typedef "Image.lvlib/Image Save File Format.ctl" = enum16{"PNG", "JPEG", "BMP"}
  T26 = typedef "AlliGator Files.lvlib/AlliGator Saved TIFF Image Type.ctl" = enum16{"Single Gate", "Sum of All Gates", "Phasor"}
  T27 = typedef "AlliGator ROIs.lvlib/AlliGator Selected ROI.ctl" = cluster{"Image Ctrl Ref":T28, "All ROIs?":bool}
  T28 = typedef "Image.lvlib/Image Control Refnum.ctl" = refnum<vi>
  T29 = typedef "Utilities.lvlib/Read-Write.ctl" = enum16{"Read", "Write"}
  T30 = typedef "AlliGator Internal Variables.lvlib/AlliGator Internal Variables v2.ctl" = cluster{"Displayed Image":T24, "White Light Image":T24, "Mask Image":T24, "ROI Mask Image":T24, "Current Dataset Images 1":T31, "Background Dataset Images 1":T31, "Current Dataset Images 2":T31, "Background Dataset Images 2":T31, "Current Dataset Arithmetic Images":T31, "Accumulated Dataset Images 1":T31, "Accumulated Dataset Images 2":T31, "Accumulated Dataset Arithmetic Images":T31, "Phasor Plot Image":T24, "Decay Fit Parameter Map Image":T24, "Single Data Point Path":path, "White Light Image Path":path, "Mask Image Path":path, "Time-Series Folder":path, "[Time-Series Paths]":path[], "Current Dataset":i32, "Single Dataset Type":T32, "Current Folder":string, "AlliGator Data Series Type":T33, "# Datasets":i32, "Dual-Channel Dataset":bool, "Selected Channel Name":string, "Dataset Channel":T34, "Channel Arithmetic":T35, "Dual-Channel Background Dataset":bool, "Background Channel":T34, "Dual-Channel Accumulated Dataset":bool, "Start Time":dbl, "[Time-Series Timestamps]":dbl[], "[Intensity Corrections]":dbl[], "Time Series Script":bool, "Type of Displayed Image":T36, "Gate Image Slide":u16, "# Gates":i32, "ROIs":T37[], "ROI Decay":cluster{"t Array":dbl[], "I Array":dbl[]}, "Valid Decay":bool, "Decay  Metadata":T38, "Reference Decay Plot Name":string, "Reference Decay":cluster{"t Array":dbl[], "I Array":dbl[]}, "Decay Shift Plot":cluster{"Time Stamps":dbl[], "Decay Shifts":dbl[]}, "[Decays Max Values]":sgl[], "[Decays Min Values]":sgl[], "Calibration Phasor":T44, "Calibration Phasor Series":T45, "Phasor Calibration Map":T46, "Calibration Map MD5 Digest":string, "Last Raw Phasor":T47, "Last Calibrated Phasor":T47, "Last Calibrated Phasor SDV":T47, "Phasor Graph:Phasor Plot":cluster{"g Array":dbl[], "s Array":dbl[]}, "Phasor Graph:Phasor SDV Plot":cluster{"g Array":dbl[], "s Array":dbl[]}, "[Phasor Graph:Raw Phasor Plots]":T48[], "Phasor Plot locked to Ref 1":i32, "[Phasor Plot(s) locked to Ref 1]":i32[], "[Phasor Plot(s) locked to Ref 2]":i32[], "[Pixel Phasors]":T47[], "[[Sum Image]]":dbl[][], "[[CSG Phasors]]":csg[][], "[[Valid Pixel?]]":bool[][], "I/m/phi Dataset":cluster{"I/m/phi Dataset?":bool, "Base Frequency":dbl[unit], "Harmonic Orders":u8[]}, "Multi Phasor Plot Data":T50, "Decay Fit Options & Parameters":T52, "Fit Options: Decay Preprocessing Parameters":T63, "Fit Options: Reference Decay":cluster{"t Array":dbl[], "I Array":dbl[]}, "Is Full Image Parameters Map":bool, "Is Single-Pixels Parameters Map":bool, "NLSF Parameters Map X Resolution":i32, "NLSF Parameters Map Y Resolution":i32, "[Single Decay Fit Parameters]":dbl[], "Fit Model":T54, "[[Multiple Decays Fit Parameters]]":dbl[][], "[[Multiple Decays Fit Parameter SDVs]]":dbl[][], "[[IRFs]]":dbl[][], "IRF Array Time Axis":dbl[], "Decay Array Time Axis":dbl[], "[Decay Fit Parameter Names]":T64[], "[[Phasor Ratios]]":dbl[][], "[[Average Lifetimes]]":dbl[][], "Amplitude Weighted Average Lifetime":bool, "[Decay Sum]":dbl[], "Parameter Maps":T65[], "[[User-defined Quantities]]":dbl[][], "User-defined Quantity":string}
  T31 = typedef "AlliGator Internal Variables.lvlib/AlliGator Gate Image Set.ctl" = cluster{"SGL Image Max":T24, "SGL Image Sum":T24, "SGL Gate Images":T24[], "SGL Image Min":T24}
  T32 = typedef "AlliGator Files.lvlib/AlliGator FLI Dataset Type.ctl" = enum16{"HDF5 FLI Dataset", "Gate Image Folder", ".sdt FLI Dataset (Becker & Hickl)", ".ptu FLI Dataset (PicoQuant)", "SS1 FLI Dataset", "SS2 FLI Dataset", "I/m/phi Dataset", ".bin FLI Dataset (PicoQuant Binned)", ".bin FLI Dataset (Piccolo Binned)"}
  T33 = typedef "AlliGator Files.lvlib/AlliGator Data Series Type.ctl" = enum16{"Not a Supported Series", "Gate Images Folder Series", "SwissSPAD 2 Dataset Series", "B&H FLI Dataset Series", "PicoQuant PTU FLI Dataset Series", "PicoQuant BIN FLI Dataset Series", "Piccolo hist BIN FLI Dataset Series", "HDF5 FLI Dataset Series"}
  T34 = typedef "AlliGator Dual-Channel Datasets.lvlib/AlliGator Dataset Channel.ctl" = enum16{"G2", "INT"}
  T35 = typedef "AlliGator Settings.lvlib/AlliGator Gate Arithmetic.ctl" = enum16{"None", "INT-G2", "G2/INT*<INT>", "(1 - G2/INT)*<INT>"}
  T36 = typedef "AlliGator Source Image.lvlib/AlliGator Displayed Image.ctl" = enum16{"Single Gate", "Sum of All Gates", "Max of All Gates", "Min of All Gates", "-", "White Ligth Image", "Mask Image"}
  T37 = typedef "Image.lvlib/Named ROI Description.ctl" = cluster{"ROI Descriptor":T22, "ROI Name":string, "Overlay Color":u32}
  T38 = typedef "AlliGator Phasor Graph.lvlib/AlliGator Decay Metadata v3.ctl" = cluster{"ROI Descriptor":T22, "ROI Center":cluster{"X":i32, "Y":i32}, "Decay Background Subtraction Info":T39, "Decay Reverted":bool, "Decay Smoothened":bool, "Decay Straightened":bool, "Fitted Tau (Decay Straightening)":dbl, "Decay Shift Parameters":T41, "Decay Shifted":bool, "Decay Extrapolated":bool, "Decay Extrapolation Parameters":T43, "Decay Normalized":bool, "Fold Decay":bool, "# Folds":u32}
  T39 = typedef "AlliGator Decay Analysis.lvlib/AlliGator Decay Preprocessing.lvlib/AlliGator Decay Background Subtraction Info.ctl" = cluster{"Laser Period":dbl[unit], "Gate Duration":dbl[unit], "Baseline Subtraction Method":T40, "Background Definition Range":cluster{"Min Gate":dbl[unit], "Max Gate":dbl[unit]}, "Total Intensity w/o Bkgd Subtraction":dbl, "Bkgd-subtracted Intensity (exp)":dbl, "# Data Points":i32, "Background/Gate":dbl, "Fitted Lifetime":dbl[unit], "Bkgd-subtracted Intensity (theo)":dbl}
  T40 = typedef "AlliGator Decay Analysis.lvlib/AlliGator Decay Preprocessing.lvlib/AlliGator Baseline Subtraction Method.ctl" = enum16{"Mean", "Min", "Square Gated Single-Exponential", "File", "Constant"}
  T41 = typedef "XY Graph Add-Ons.lvlib/XY Graph Plot Shift Parameters.ctl" = cluster{"Type":T42, "Shift":dbl[unit], "Threshold":dbl, "Rotate":bool}
  T42 = typedef "XY Graph Add-Ons.lvlib/XY Graph Plot Shift Method.ctl" = enum16{"Default", "CFD", "Threshold", "Cross-Correlation"}
  T43 = typedef "AlliGator Decay Analysis.lvlib/AlliGator Decay Preprocessing.lvlib/AlliGator Decay Extrapolation Parameters.ctl" = cluster{"Additional Points":u32, "Head Fraction":dbl, "Fitted Tau":dbl, "Use Periodicity":bool, "Use Cursors":bool, "Tail Fraction":dbl}
  T44 = typedef "Phasor.lvlib/Calibration Phasor (m, phi).ctl" = cluster{"m":dbl, "phi":dbl, "Phasor Frequency":dbl[unit], "Reference Lifetime":dbl[unit]}
  T45 = typedef "Phasor.lvlib/Phasor Reference Series.ctl" = cluster{"m Array":dbl[], "phi Array":dbl[], "Phasor Frequency":dbl[unit], "Calibration Lifetime":dbl[unit]}
  T46 = typedef "Phasor.lvlib/Phasor Calibration Map v2.ctl" = cluster{"Phasor Frequency":dbl[unit], "Calibration Lifetime":dbl[unit], "ROI Centers":cluster{"X":i32, "Y":i32}[], "ROI Descriptors":T22[], "Map Resolution X":i32, "Map Resolution Y":i32, "z Array":cdb[]}
  T47 = typedef "Phasor.lvlib/Phasor (g, s).ctl" = cluster{"g":dbl, "s":dbl}
  T48 = typedef "AlliGator Phasor Graph.lvlib/AlliGator Raw Phasor Plot Data v4.ctl" = cluster{"Phasor Plot Name":string, "Raw Phasor Plot":T47[], "Phasor Frequency":dbl[unit], "[Decay Metadata]":T38[], "Raw Phasor Plot SDV":T47[], "Phasor SDV Options":T49, "[Calibration Phasor]":T44[]}
  T49 = typedef "Phasor.lvlib/Phasor Standard Deviation Options.ctl" = cluster{"Compute Estimated SDV":bool, "# Replicas":u32, "Use Estimated Average Phasor":bool}
  T50 = typedef "AlliGator Phasor Plot.lvlib/AlliGator Phasor Multi-Harmonic Data.ctl" = cluster{"Base Frequency":dbl[unit], "# Harmonics":u8, "Harmonic Orders":u8[], "Phasor Plot Settings Checksum":u64, "Phasor Harmonic Data Array":T51[]}
  T51 = typedef "Phasor.lvlib/Phasor Harmonic Data.ctl" = cluster{"Phasor Harmonic Name":string, "Phasor Plot Settings Checksum":u64, "Phasor Frequency":dbl[unit], "Base Frequency":dbl[unit], "Harmonic Order":u8, "Phasor Plot Parameters":string, "Phasor Array [[CSG]]":csg[][], "Dataset File Path":path}
  T52 = typedef "AlliGator Decay Fit Parameter Map.lvlib/AlliGator Decay Fit Options & Parameters v2.ctl" = cluster{"SYNC Period":dbl[unit], "Fit Options":T53, "Fit Parameter Constraints":T60[], "MLE Baseline Offset":dbl, "MLE Baseline Offset Type":T62}
  T53 = typedef "Fits.lvlib/Decay Fit Options v2.ctl" = cluster{"Show Fit Residuals":bool, "Fit Model":T54, "Residual Type":T55, "Max Decay Percentile":dbl, "Min Decay Percentile":dbl, "Show Full Decay":bool, "Weights":T56, "Fitting Method":T57, "Compute Parameter Uncertainties":bool, "Periodic Boundaries":bool, "Model Calculation":T58, "Period":dbl[unit], "Termination Criteria":cluster{"Max Iterations":i32, "Max Function Calls":i32, "Max Time":dbl[unit], "Function Tolerance":dbl, "Parameter Tolerance":dbl, "Gradient Tolerance":dbl, "Min Lambda":dbl, "Max Lambda":dbl, "Initial Tick Count":u32}, "Offset Resolution":dbl[unit], "Use Local IRF":bool, "Fitting Algorithm":T59}
  T54 = typedef "Fits.lvlib/Decay Model.ctl" = enum16{"1-Exponential", "2-Exponentials"}
  T55 = typedef "Fits.lvlib/Residual Type.ctl" = enum16{"Standard", "Normalized", "Reduced"}
  T56 = typedef "Fits.lvlib/Fit Weights Type.ctl" = enum16{"Unweighted", "1/Variance", "Best of All"}
  T57 = typedef "Fits.lvlib/Non-linear Fitting Method v2.ctl" = enum16{"Least Square", "Least Absolute Residual", "Bisquare", "MLE", "-", "Best of All"}
  T58 = typedef "Fits.lvlib/Fit Calculation Method.ctl" = enum16{"Simulation", "Convolution", "Integration"}
  T59 = typedef "Fits.lvlib/Non-linear Fitting Algorithm.ctl" = enum16{"Levenberg-Marquardt", "Trust-Region Dogleg"}
  T60 = typedef "AlliGator Decay Analysis.lvlib/AlliGator Decay Fit.lvlib/AlliGator Decay Fit Parameter Constraints 2.ctl" = cluster{"Fit Parameter":T61, "Min Value":dbl, "Max Value":dbl, "Global":bool, "Used":bool}
  T61 = typedef "Fits.lvlib/Decay Fit Parameters In List.ctl" = enum16{"Offset", "Baseline", "A_1", "tau_1", "A_2", "tau_2"}
  T62 = typedef "Fits.lvlib/MLE Baseline Offset Type.ctl" = enum32{"Absolute", "Percentage"}
  T63 = typedef "AlliGator Decay Analysis.lvlib/AlliGator Decay Preprocessing.lvlib/AlliGator Decay Preprocessing Parameters.ctl" = cluster{"Background Subtraction":bool, "Straighten Decay":bool, "Reverse Gates":bool, "1-Normalized Decay":bool, "Smoothen Decay":bool, "Smoothing Parameter":dbl, "Shift Decay":bool, "Decay Shift Parameters":T41, "Extrapolate Decay":bool, "Additional Points":u32, "Head Fraction":dbl, "Pixel-Normalize Decay":bool, "Use Periodicity":bool, "Use Cursors":bool, "Tail Fraction":dbl, "Use Decay Pre-Processing":bool, "Fold Decay":bool, "# Folds":u32, "[0-1]-Normalized Decay":bool}
  T64 = typedef "Fits.lvlib/Decay Fit Parameters & Derived Quantities List.ctl" = enum16{"Offset", "Baseline", "A_1", "tau_1", "A_2", "tau_2", "<tau>_a", "f1_a", "f2_a", "<tau>_i", "f1_i", "f2_i", "-", "R^2", "Chi^2"}
  T65 = typedef "AlliGator Parameter Maps Data.ctl" = cluster{"Map Set Name":string, "[Parameter Names]":string[], "[[Parameters]]":dbl[][], "[[Parameter SDVs]]":dbl[][], "Decay Array Time Axis":dbl[], "[[IRFs]]":dbl[][], "IRF Array Time Axis":dbl[]}
  T66 = typedef "Image.lvlib/Image ROI Statistics Selection.ctl" = cluster{"Area (pixels)":bool, "% of Image":bool, "Total Intensity":bool, "Mean Intensity":bool, "Median Intensity":bool, "Mode Intensity":bool, "Intensity Standard Deviation":bool, "Min Intensity":bool, "Max Intensity":bool, "Mean SNR":bool, "Median SNR":bool, "Mode SNR":bool, "SNR Standard Deviation":bool, "Max SNR":bool, "Min SNR":bool, "# Rejected Pixels (NaN, Inf)":bool, "# Negative Pixels":bool, "Long Axis Length":bool, "Short Axis Length":bool, "Aspect Ratio":bool}
  T67 = cluster{"Global Rectangle":i32[], "Contours":cluster{"Contour Type":u32, "ROI Type":u32, "Points":i32[]}[]}
  T68 = typedef "Image.lvlib/Image Control ROI Description v2.ctl" = cluster{"Image Control Label":string, "Named ROI Description":T37}
  T69 = typedef "Image.lvlib/Image Display User Event Data.ctl" = cluster{"Image Control Refnum":T28, "Coords":T70, "button info":cluster{"button 1":bool, "button 2":bool, "button 3":bool, "button 4":bool}, "keys pressed":enum16{"0", "1", "2", "3", "4", "5", "6", "7", "8", "9", "A", "B", "C", "D", "E", "F", "G", "H", "I", "J", "K", "L", "M", "N", "O", "P", "Q", "R", "S", "T", "U", "V", "W", "X", "Y", "Z", "F1", "F2", "F3", "F4", "F5", "F6", "F7", "F8", "F9", "F10", "F11", "F12", "F13", "F14", "F15", "ADD", "BACK", "BACKSLASH", "CAPITAL", "COMMA", "DECIMAL", "DELETE", "DIVIDE", "DOWN", "END", "EQUALS", "ESCAPE", "GRAVE (`)", "HOME", "INSERT", "LBRACKET", "LCONTROL", "LEFT", "L ALT", "LSHIFT", "LWIN", "MINUS", "MULTIPLY", "NEXT", "NUMLOCK", "NUMPAD_0", "NUMPAD_1", "NUMPAD_2", "NUMPAD_3", "NUMPAD_4", "NUMPAD_5", "NUMPAD_6", "NUMPAD_7", "NUMPAD_8", "NUMPAD_9", "PAUSE", "PERIOD", "PRIOR (PG UP)", "RBRACKET", "RCONTROL", "RETURN", "RIGHT", "R ALT", "RSHIFT", "RWIN", "SCROLL", "SEMICOLON", "SLASH", "SPACE", "SUBTRACT", "TAB", "UP", "ENTER (num pad)", "' (quote)"}[]}
  T70 = typedef "LVPoint32TypeDef.ctl" = cluster{"Horizontal":i32, "Vertical":i32}
  T71 = typedef "AlliGator Phasor Plot.lvlib/AlliGator Phasor Plot Mouse Up Event Data.ctl" = cluster{"Current ROI Tool":u32, "ROI Descriptor":T72, "Shift":bool, "Alt":bool}
  T72 = typedef "Image.lvlib/Image ROI Descriptor.ctl" = cluster{"Global Rectangle":i32[], "Contours":T73[]}
  T73 = typedef "Image.lvlib/Image Contour Definition.ctl" = cluster{"Contour Type":T74, "ROI Type":T75, "Points":i32[]}
  T74 = typedef "Image.lvlib/Image Contour ID.ctl" = enum32{"External", "Internal"}
  T75 = typedef "Image.lvlib/Image ROI Type.ctl" = enum16{"No Selection", "Point", "Line", "Rectangle", "Oval", "Polygon", "Freehand Region", "Annulus", "Unused2", "Unused3", "Broken Line", "Freehand Line", "Rotated Rectangle"}
  T76 = typedef "Image.lvlib/Image Display Event.ctl" = cluster{"Item Tag":string, "Image Control Refnum":T28, "Coords":T70, "Item Path":string}
  T77 = typedef "AlliGator ROIs.lvlib/AlliGator ROI Selection Data.ctl" = cluster{"Action":T21, "ID":i32}
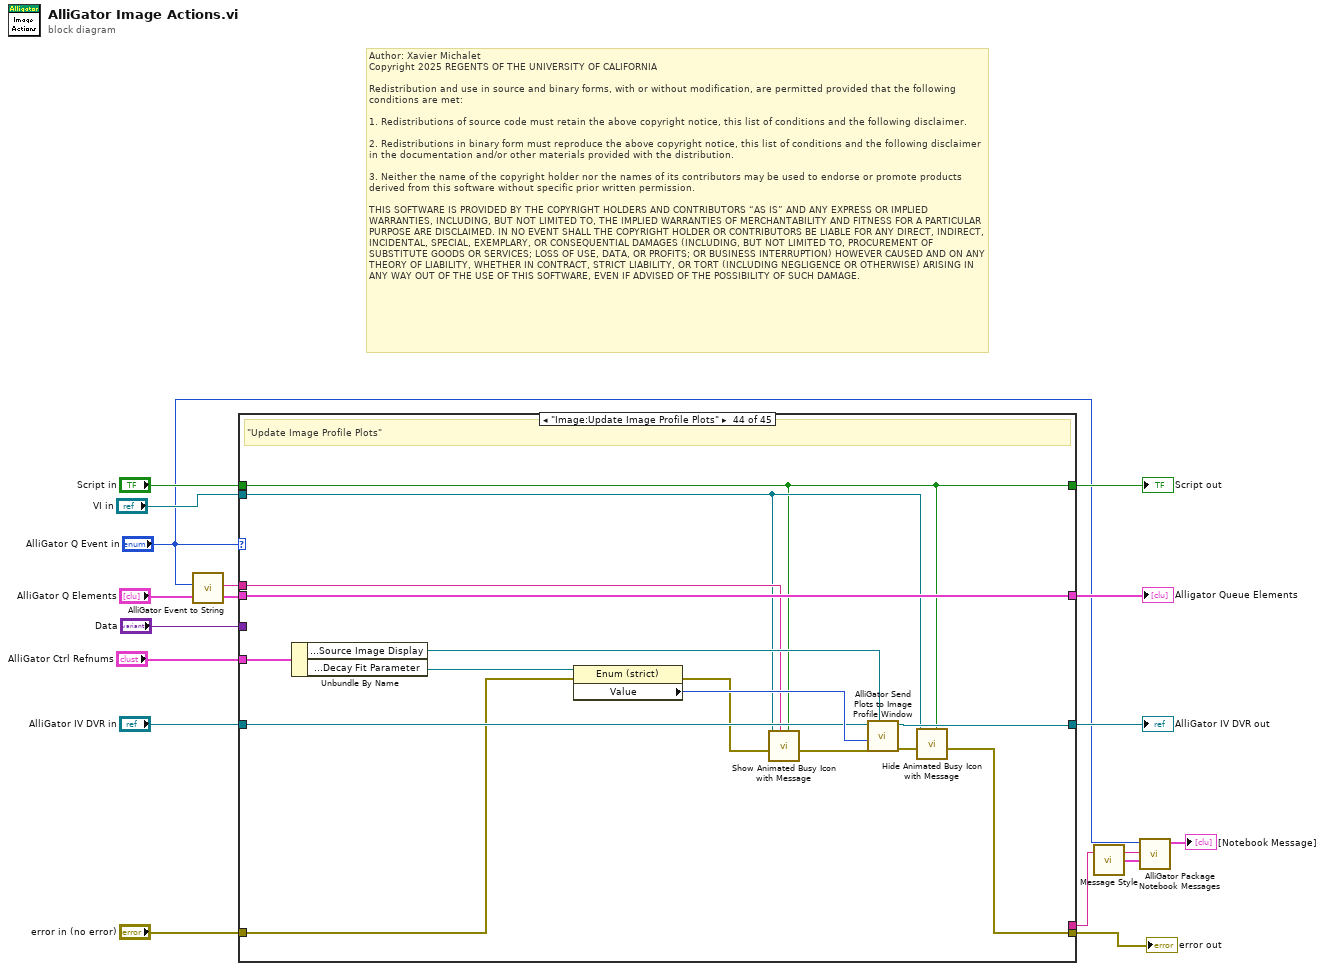
[diagram p0: block diagram]
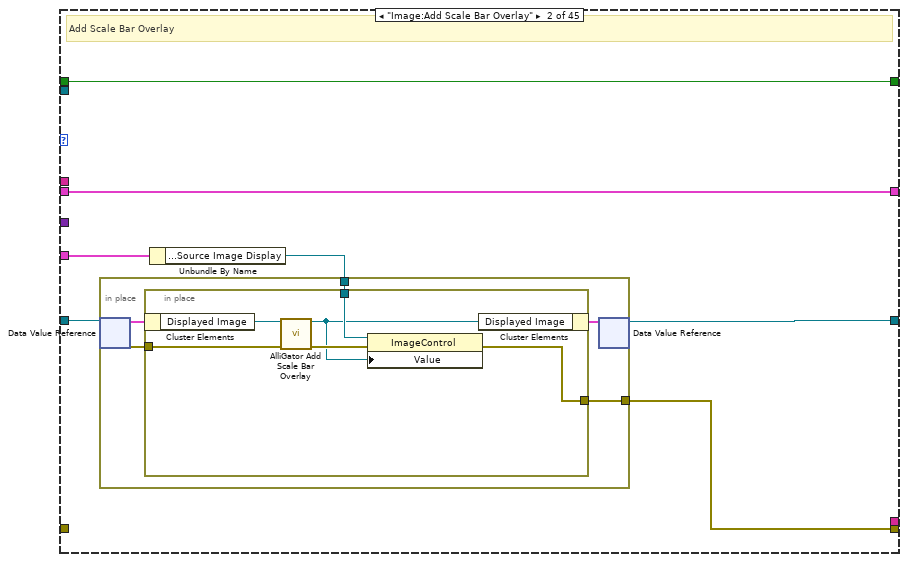
[diagram p3: hidden frame]
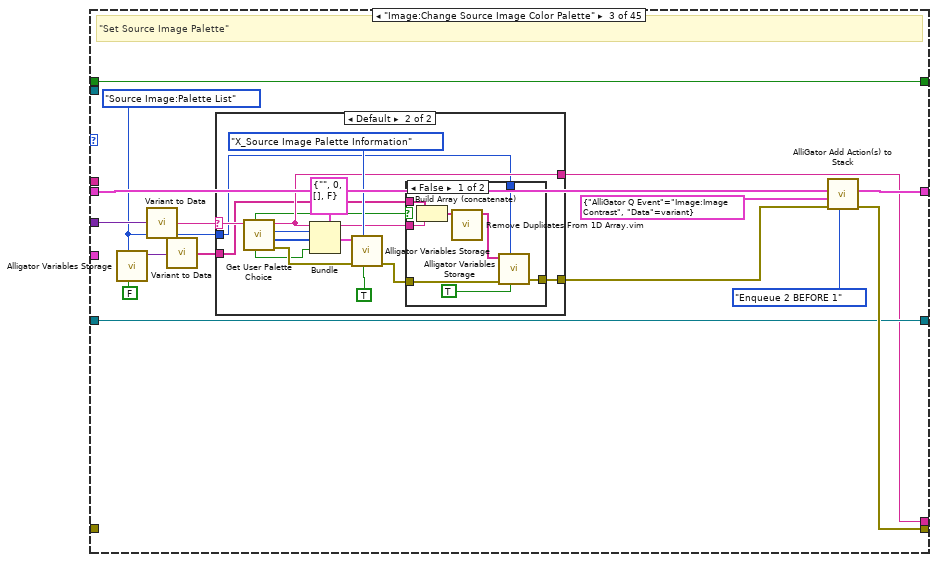
[diagram p4: hidden frame]
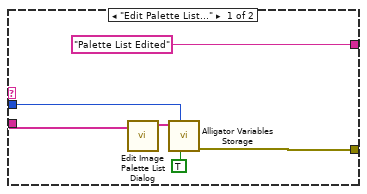
[diagram p5: hidden frame]
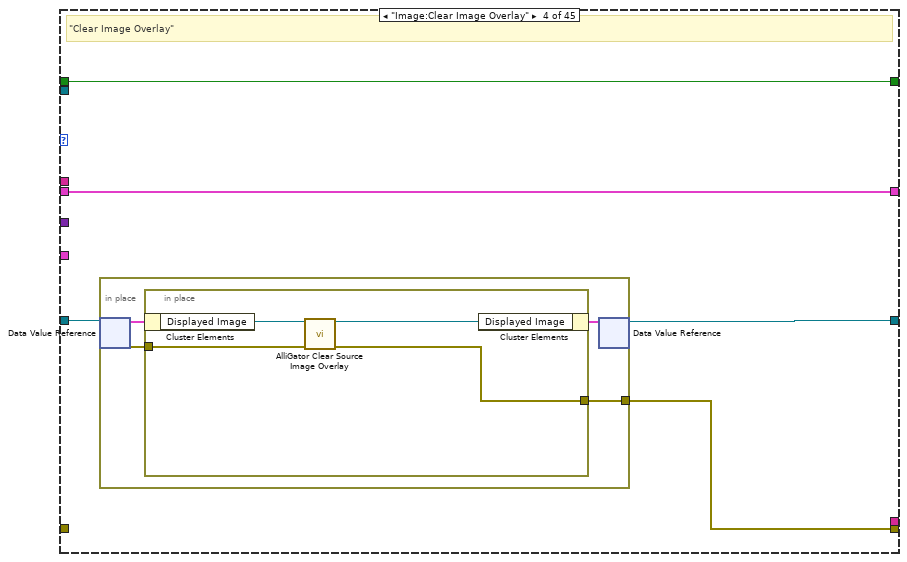
[diagram p7: hidden frame]
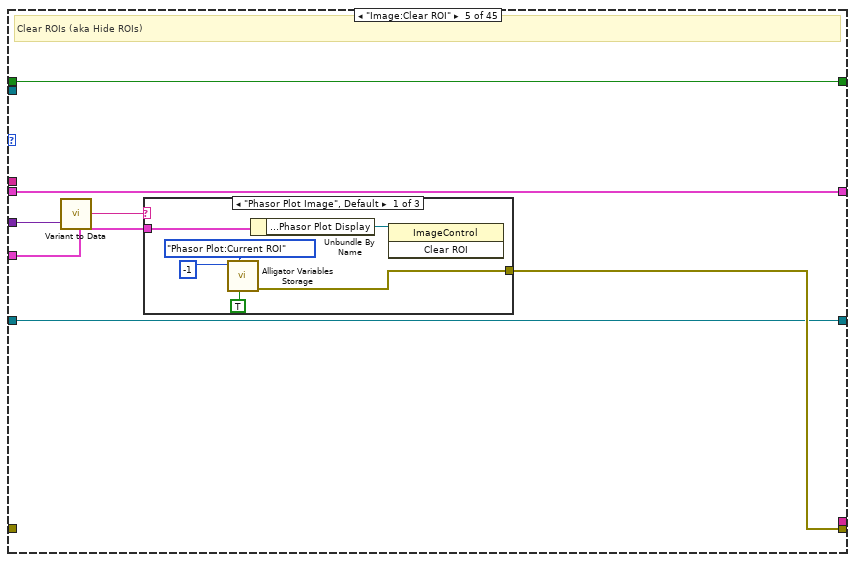
[diagram p8: hidden frame]
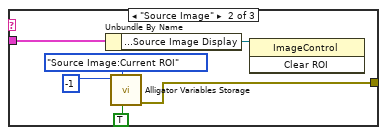
[diagram p9: hidden frame]
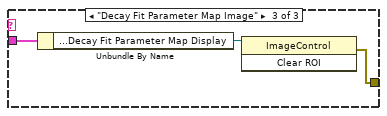
[diagram p10: hidden frame]
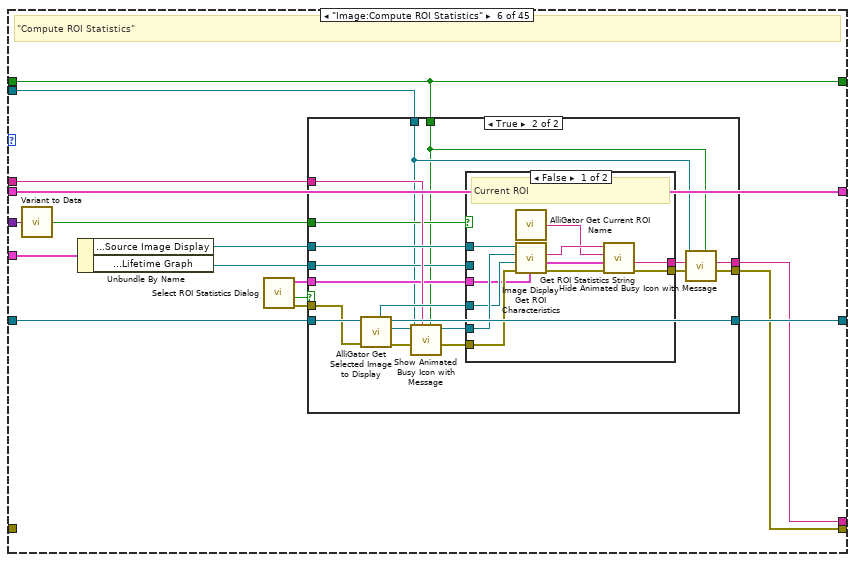
[diagram p11: hidden frame]
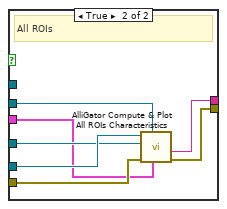
[diagram p13: hidden frame]
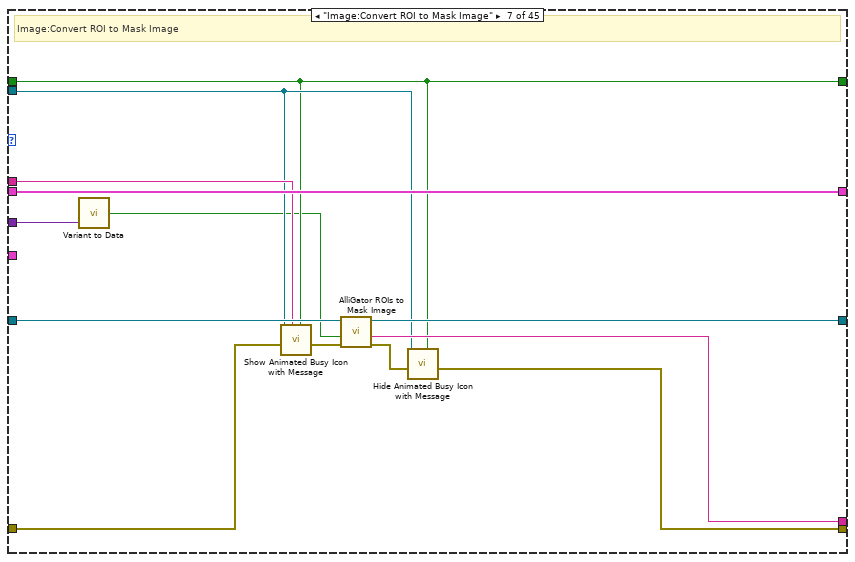
[diagram p14: hidden frame]
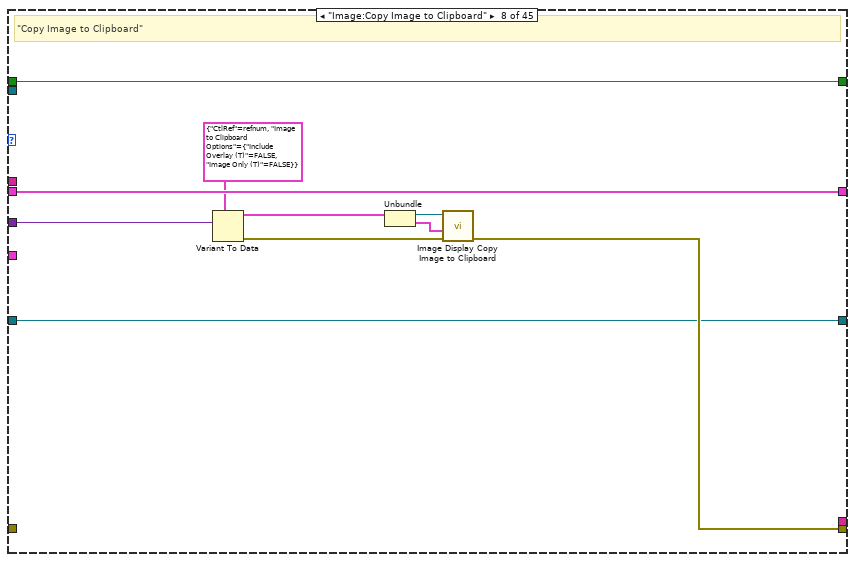
[diagram p15: hidden frame]
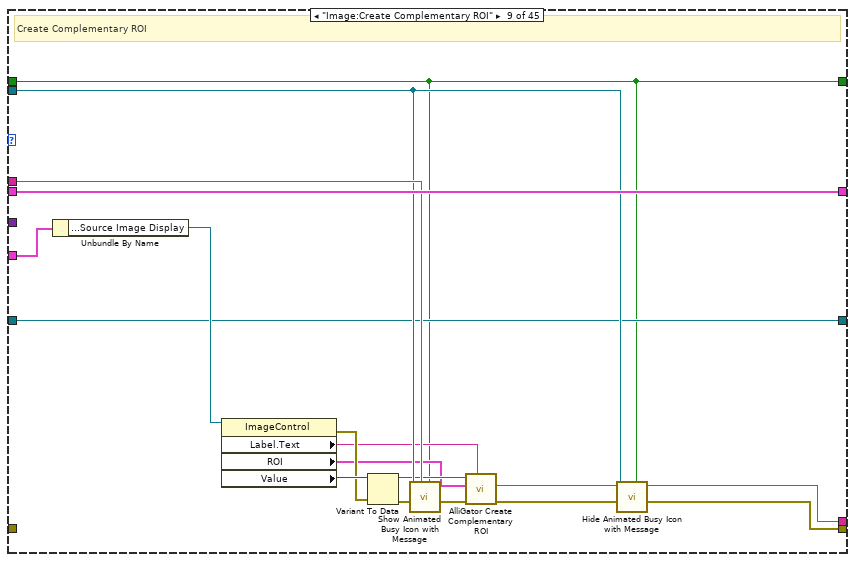
[diagram p16: hidden frame]
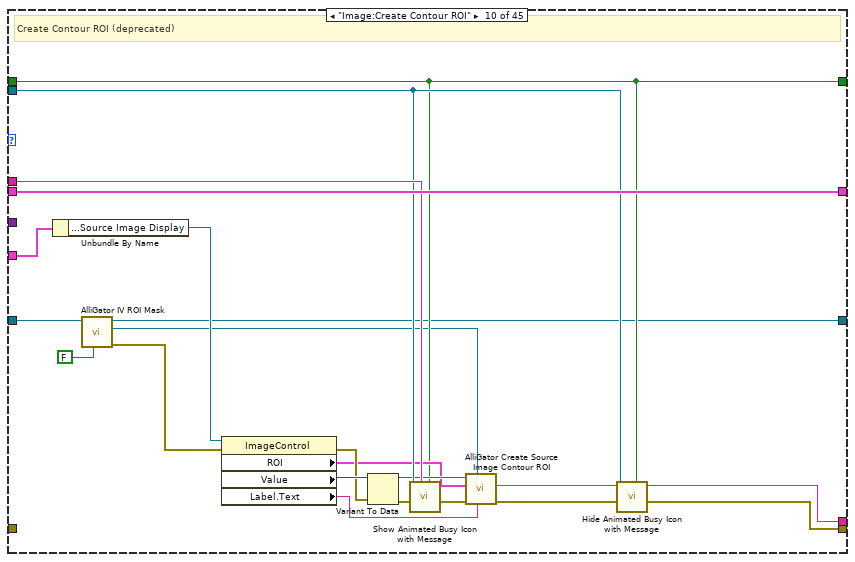
[diagram p17: hidden frame]
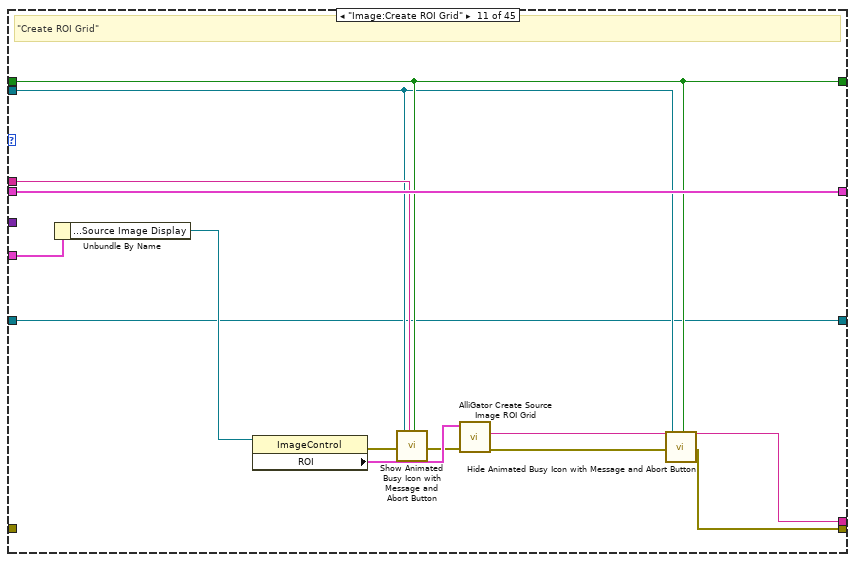
[diagram p18: hidden frame]
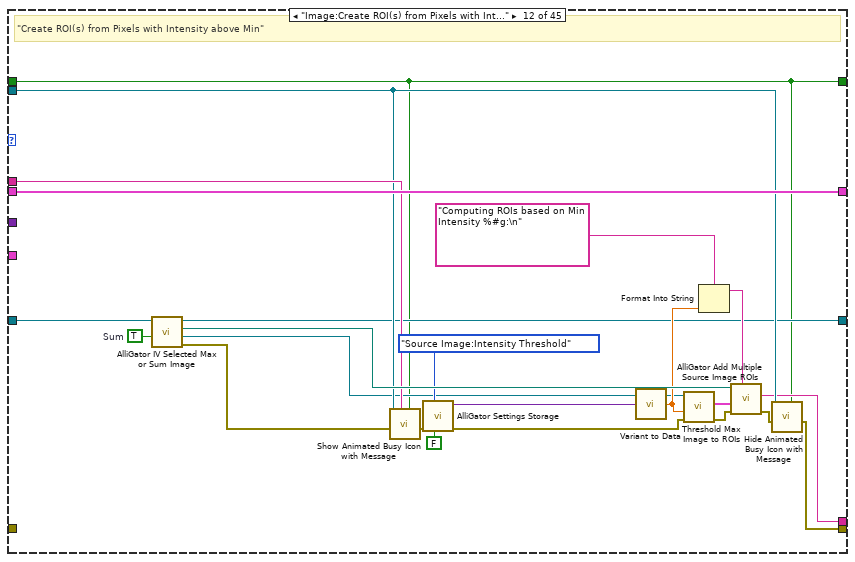
[diagram p19: hidden frame]
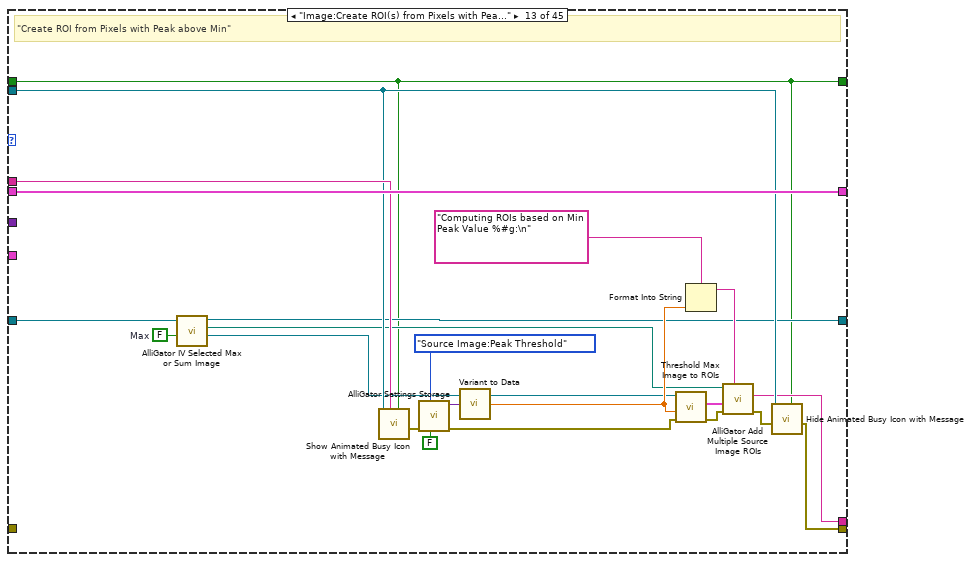
[diagram p20: hidden frame]
diagram:
  # "Author: Xavier Michalet\nCopyright 2025 REGENTS OF THE UNIVERSITY OF CALIFORNIA\n\nRedistribution and use in source and binary forms, with or without modification, are permitted provided that the following conditions are met:\n\n1. Redistributions of source code must retain the above copyright notice, this list of conditions and the following disclaimer.\n\n2. Redistributions in binary form must reproduce the above copyright notice, this list of conditions and the following disclaimer in the documentation and/or other materials provided with the distribution.\n\n3. Neither the name of the copyright holder nor the names of its contributors may be used to endorse or promote products derived from this software without specific prior written permission.\n\nTHIS SOFTWARE IS PROVIDED BY THE COPYRIGHT HOLDERS AND CONTRIBUTORS “AS IS” AND ANY EXPRESS OR IMPLIED WARRANTIES, INCLUDING, BUT NOT LIMITED TO, THE IMPLIED WARRANTIES OF MERCHANTABILITY AND FITNESS FOR A PARTICULAR PURPOSE ARE DISCLAIMED. IN NO EVENT SHALL THE COPYRIGHT HOLDER OR CONTRIBUTORS BE LIABLE FOR ANY DIRECT, INDIRECT, INCIDENTAL, SPECIAL, EXEMPLARY, OR CONSEQUENTIAL DAMAGES (INCLUDING, BUT NOT LIMITED TO, PROCUREMENT OF SUBSTITUTE GOODS OR SERVICES; LOSS OF USE, DATA, OR PROFITS; OR BUSINESS INTERRUPTION) HOWEVER CAUSED AND ON ANY THEORY OF LIABILITY, WHETHER IN CONTRACT, STRICT LIABILITY, OR TORT (INCLUDING NEGLIGENCE OR OTHERWISE) ARISING IN ANY WAY OUT OF THE USE OF THIS SOFTWARE, EVEN IF ADVISED OF THE POSSIBILITY OF SUCH DAMAGE."
  n1 = call "AlliGator Event to String.vi"("AlliGator Q Event"="AlliGator Q Event in") -> ("String"=w6:string)  [unwired: 8 in]
  n2 = case shown="\"Image:Update Image Profile Plots\"" "AlliGator Q Event in" {
    tunnel: "Data" -> [_ _ w53 _ w102 w124 w179 w192 _ _ _ _ _ _ _ _ _ _ w369 w389 w398 _ w452 w516 _ w532 w546 _ _ w594 w610 w661 w682 w726 w766 w808 w812 _ w832 _ w863 w879 _ _ _]
    tunnel: "AlliGator Q Elements" -> [w20 w27 w52 w88 w103 w134 w183 w193 w210 w231 w244 w267 w289 w299 w309 w317 w333 w347 w370 w393 w428 w448 w462 w517 w527 w534 w544 w555 w569 w589 w620 w665 w703 w729 w781 w809 w816 w829 w836 w848 w857 w883 w893 w908 w915]
    tunnel: [w20 w27 w51 w88 w103 w134 w183 w193 w210 w231 w244 w267 w289 w296 w306 w317 w330 w347 w370 w393 w428 w446 w462 w517 w524 w533 w543 w555 w569 w588 w620 w665 w703 w729 w781 w809 w816 w829 w836 w848 w855 w883 w890 w908 w915] -> w8
    tunnel: "VI in" -> [_ _ _ _ _ w126 w173 _ w204 w225 w234 w252 w275 _ _ _ _ w335 _ w382 w410 _ w461 w508 _ _ _ _ _ w590 w608 w641 w684 w719 w752 w795 _ _ _ w846 w859 _ _ w895 _]
    tunnel: [w19 w26 w46 w87 w100 w125 w172 w186 w194 w216 w238 w245 w268 w298 w308 w316 w332 w334 w362 w381 w403 w451 w460 w505 w526 w536 w548 w554 w568 w578 w599 w640 w683 w711 w751 w794 w815 w824 w835 w845 w858 w882 w892 w894 w914] -> w9
    tunnel: "Script in" -> [w19 w26 w46 w87 w100 w125 w172 w186 w194 w216 w238 w245 w268 w298 w308 w316 w332 w334 w362 w381 w403 w451 w460 w505 w526 w536 w548 w554 w568 w578 w599 w640 w683 w711 w751 w794 w815 w824 w835 w845 w858 w882 w892 w894 w914]
    tunnel: w6 -> [_ _ _ _ _ w128 w175 _ w208 w229 w236 w263 w285 _ _ _ _ w339 _ w384 w409 _ w455 w503 _ _ _ _ _ w591 w614 w643 w685 w718 w753 w797 _ _ _ w844 _ _ _ w896 _]
    tunnel: "error in (no error)" -> [w18 _ _ _ _ _ w177 _ _ _ _ _ _ w291 w301 w311 w325 w341 _ w386 _ w450 _ w504 w519 w528 w545 w549 _ _ _ _ _ _ _ w790 w814 _ w834 w847 _ _ w885 w899 _]
    tunnel: [w18 w23 w45 w84 w99 w127 w174 w185 w206 w227 w239 w264 w286 w290 w300 w312 w324 w336 w361 w383 w427 w450 w459 w510 w518 w529 w542 w550 w561 w585 w612 w645 w693 w727 w761 w796 w814 w820 w834 w847 w849 w873 w884 w897 w913] -> w5
    tunnel: "AlliGator Ctrl Refnums" -> [_ w22 _ _ w98 w132 _ _ w207 w228 w235 _ _ _ _ _ _ _ w357 _ w411 _ w457 _ _ _ w539 w551 w560 _ w613 w651 w695 _ w763 w793 _ w819 _ w839 w853 w875 _ w906 w911]
    tunnel: "AlliGator IV DVR in" -> [w17 w25 w44 w86 w97 w131 w181 w184 w202 w223 w233 w249 w274 w297 w307 w315 w331 w345 w360 w391 w408 w449 w454 w507 w525 w535 w547 w553 w557 w583 w605 w648 w669 w710 w750 w800 w813 w818 w833 w843 w861 w865 w891 w903 w910]
    tunnel: [w17 w24 w44 w85 w97 w130 w180 w184 w202 w214 w233 w250 w272 w297 w307 w315 w331 w344 w360 w390 w407 w449 w453 w507 w525 w535 w547 w552 w557 w582 w603 w647 w668 w709 w747 w800 w813 w818 w833 w842 w861 w865 w891 w902 w910] -> w16
    tunnel: [_ _ w43 _ _ w129 w178 _ w201 w222 w232 w246 w269 _ _ w310 _ w340 w359 w387 _ _ _ w506 _ _ _ _ w556 w579 w601 w646 w688 w712 w756 w799 _ w817 _ _ _ w864 _ _ w909] -> w2
    frame "---- Image ----", Default {
    }
    frame "Image:Add Scale Bar Overlay" {
      # "Add Scale Bar Overlay"
      n3 = Unbundle By Name(w22) -> ("Registered Events Ctrl Refnums.Source Image Display"=w21:refnum<vi>)
      n4 = in-place "In Place Element Structure" {
        in-place-border: [w29] -> w23
        in-place-border: w21 -> [w28]
        n5 = in-place-dvr #1 ("Data Value Reference Read / Write Element")(w25) -> (w32:T30, w30:errorcluster)
        n6 = in-place "In Place Element Structure" {
          in-place-border: w30 -> [w37]
          in-place-border: [w34] -> w29
          in-place-border: w28 -> [w36]
          n7 = in-place-cluster #2 ("Unbundle / Bundle Elements")(w32) -> ("Displayed Image"=w38:T24)
          n8 = call "AlliGator Add Scale Bar Overlay.vi"("Source Image in"=w38, "Error In"=w37) -> ("Source Image out"=w33:T24, "Error Out"=w35:errorcluster)  [unwired: 12 in]
          n9 = property class="ImageControl"(reference=w36, error in=w35, "Value"=w33) -> (error out=w34:errorcluster)  [unwired: 1 out]
          n10 = in-place-cluster #2 ("Unbundle / Bundle Elements")("Displayed Image"=w33) -> (w31:T30)
        }
        n11 = in-place-dvr #1 ("Data Value Reference Read / Write Element")(w31) -> (w24:refnum<data-value>)  [unwired: 1 out]
      }
    }
    frame "Image:Change Source Image Color Palette" {
      w41 = AlliGator_Variables_List."Source Image:Palette List" ("Alligator Variable")
      # "\"Set Source Image Palette\""
      n12 = call "Alligator Variables Storage.vi"("Get(F)/Set"=FALSE, "AlliGator Variable"=w41) -> ("Data out"=w40:variant)  [unwired: 7 in, 2 out]
      n13 = call-poly "Variant to Data.vi"("Variant"=w53) -> ("String"=w50:string)  [unwired: 8 in]
      n14 = call-poly "Variant to Data.vi"("Variant"=w40) -> ("String Array"=w39:string[])  [unwired: 8 in]
      n15 = case shown="Default" w50 {
        selector: w50 -> [_ w74]
        tunnel: [w57 w64] -> w48
        tunnel: ["Palette List Edited" ("Append to Message") w63] -> w43
        tunnel: w41 -> [w55 w61]
        tunnel: w39 -> [w54 w62]
        frame "Edit Palette List..." {
          n16 = call "Edit Image Palette List Dialog.vi"("Palette List (in)"=w54) -> ("Palette List (out)"=w59:string[])  [unwired: 10 in]
          n17 = call "Alligator Variables Storage.vi"("Get(F)/Set"=TRUE, "AlliGator Variable"=w55, "Data in"=w59) -> ("Error Out"=w57:errorcluster)  [unwired: 6 in, 2 out]
        }
        frame Default {
          n18 = call "Get User Palette Choice.vi"("Palette"=w74) -> ("Error Out"=w68:errorcluster, "Palette Colors"=w72:u32[], "Palette Type"=w73:T17, "Palette Name (# Colors)"=w63:string, "Interpolate?"=w67:bool, "Built-in Palette?"=w60:bool)  [unwired: 3 in, 2 out]
          n19 = Bundle(cluster=T16 {"Palette Name [# Colors,int?,inv?]"="", "Palette Type"=0, "Palette Colors"=[], "Interpolate?"=FALSE} ("Image Display Palette Information"), "Palette Name [# Colors,int?,inv?]"=w63, "Palette Type"=w73, "Palette Colors"=w72, "Interpolate?"=w67) -> (w70:T16)
          n20 = call "Alligator Variables Storage.vi"("Get(F)/Set"=TRUE, "AlliGator Variable"=AlliGator_Variables_List."X_Source Image Palette Information" ("Alligator Variable"), "Error In"=w68, "Data in"=w70) -> ("Error Out"=w65:errorcluster)  [unwired: 5 in, 2 out]
          n21 = case shown="False" w60 {
            tunnel: w65 -> [w82 w83]
            tunnel: [w81 w83] -> w64
            tunnel: w63 -> [w80 _]
            tunnel: w62 -> [w79 _]
            tunnel: w61 -> [w77 _]
            frame False {
              n22 = Build Array (concatenate)(w79, w80) -> (w78:string[])
              n23 = call "Remove Duplicates From 1D Array.vim"("array"=w78) -> ("array with duplicates removed"=w76:string[])  [unwired: 10 in]
              n24 = call "Alligator Variables Storage.vi"("Get(F)/Set"=TRUE, "AlliGator Variable"=w77, "Error In"=w82, "Data in"=w76) -> ("Error Out"=w81:errorcluster)  [unwired: 5 in, 2 out]
            }
            frame True {
            }
          }
        }
      }
      n25 = call-poly "AlliGator Add Action(s) to Stack.vi"("Elements Order in Action Stack (Default: 2 BEFORE 1)"=Alligator_Elements_Order_in_Action_Stack."Enqueue 2 BEFORE 1", "Error In"=w48, "Alligator Atomic Action"=T4 {"AlliGator Q Event"=enum."Image:Image Contrast", "Data"=variant}, "Alligator Queue Element 1"=w52) -> ("Error Out"=w45:errorcluster, "Alligator Queue Element 1 (+ 2)"=w51:T4[])  [unwired: 6 in]
    }
    frame "Image:Clear Image Overlay" {
      # "\"Clear Image Overlay\""
      n26 = in-place "In Place Element Structure" {
        in-place-border: [w89] -> w84
        n27 = in-place-dvr #3 ("Data Value Reference Read / Write Element")(w86) -> (w92:T30, w90:errorcluster)
        n28 = in-place "In Place Element Structure" {
          in-place-border: w90 -> [w94]
          in-place-border: [w93] -> w89
          n29 = in-place-cluster #4 ("Unbundle / Bundle Elements")(w92) -> ("Displayed Image"=w96:T24)
          n30 = call "AlliGator Clear Source Image Overlay.vi"("Source Image in"=w96, "Error In"=w94) -> ("Source Image out"=w95:T24, "Error Out"=w93:errorcluster)  [unwired: 12 in]
          n31 = in-place-cluster #4 ("Unbundle / Bundle Elements")("Displayed Image"=w95) -> (w91:T30)
        }
        n32 = in-place-dvr #3 ("Data Value Reference Read / Write Element")(w91) -> (w85:refnum<data-value>)  [unwired: 1 out]
      }
    }
    frame "Image:Clear ROI" {
      # "Clear ROIs (aka Hide ROIs)"
      n33 = call-poly "Variant to Data.vi"("Variant"=w102) -> ("String"=w101:string)  [unwired: 8 in]
      n34 = case shown="\"Phasor Plot Image\", Default" w101 {
        tunnel: [w106 w112 w116] -> w99
        tunnel: w98 -> [w105 w110 w117]
        frame "Phasor Plot Image", Default {
          n35 = call "Alligator Variables Storage.vi"("Get(F)/Set"=TRUE, "AlliGator Variable"=AlliGator_Variables_List."Phasor Plot:Current ROI" ("Alligator Variable"), "Data in"=-1 ("Current ROI")) -> ("Error Out"=w106:errorcluster)  [unwired: 6 in, 2 out]
          n36 = Unbundle By Name(w105) -> ("Registered Events Ctrl Refnums.Phasor Plot Display"=w104:refnum<vi>)
          n37 = invoke on="Invoke Node" class="ImageControl" method="Clear ROI"(reference=w104) -> ()  [unwired: 2 in, 3 out]
        }
        frame "Source Image" {
          n38 = Unbundle By Name(w110) -> ("Registered Events Ctrl Refnums.Source Image Display"=w111:refnum<vi>)
          n39 = call "Alligator Variables Storage.vi"("Get(F)/Set"=TRUE, "AlliGator Variable"=AlliGator_Variables_List."Source Image:Current ROI" ("Alligator Variable"), "Data in"=-1 ("Current ROI")) -> ("Error Out"=w112:errorcluster)  [unwired: 6 in, 2 out]
          n40 = invoke on="Invoke Node" class="ImageControl" method="Clear ROI"(reference=w111) -> ()  [unwired: 2 in, 3 out]
        }
        frame "Decay Fit Parameter Map Image" {
          n41 = Unbundle By Name(w117) -> ("Registered Events Ctrl Refnums.Decay Fit Parameter Map Display"=w118:refnum<vi>)
          n42 = invoke on="Invoke Node" class="ImageControl" method="Clear ROI"(reference=w118) -> (error out=w116:errorcluster)  [unwired: 2 in, 2 out]
        }
      }
    }
    frame "Image:Compute ROI Statistics" {
      # "\"Compute ROI Statistics\""
      n43 = call-poly "Variant to Data.vi"("Variant"=w124) -> ("Value"=w123:bool)  [unwired: 8 in]
      n44 = Unbundle By Name(w132) -> ("Registered Events Ctrl Refnums.Source Image Display"=w133:refnum<vi>, "Registered Events Ctrl Refnums.Lifetime Graph"=w122:refnum<vi>)
      n45 = call "Select ROI Statistics Dialog.vi"() -> ("error out"=w119:errorcluster, "OK?"=w121:bool, "ROI Statistics out"=w120:T66)  [unwired: 9 in]
      n46 = case shown="True" w121 {
        tunnel: w133 -> [_ w151]
        tunnel: w131 -> [w135 w149]
        tunnel: [w135 w148] -> w130
        tunnel: [_ w145] -> w129
        tunnel: w128 -> [_ w143]
        tunnel: [_ w142] -> w127
        tunnel: w126 -> [_ w137]
        tunnel: w125 -> [_ w136]
        tunnel: w123 -> [_ w141]
        tunnel: w122 -> [_ w140]
        tunnel: w120 -> [_ w138]
        tunnel: w119 -> [_ w139]
        frame False {
        }
        frame True {
          n47 = call "AlliGator Get Selected Image to Display.vi"("Error In"=w139, "AlliGator IV DVR in"=w149) -> ("Error Out"=w147:errorcluster, "Image out"=w150:T24, "AlliGator IV DVR out"=w148:refnum<data-value>, "ROI Mask"=w146:T24)  [unwired: 4 in, 2 out]
          n48 = call "Show Animated Busy Icon with Message.vi"("Already active? (F)"=w136, "Message"=w143, "Error In"=w147, "Target VI Refnum"=w137) -> ("Error Out"=w144:errorcluster)  [unwired: 7 in]
          n49 = case shown="False" w141 {
            tunnel: [w162 w169] -> w152
            tunnel: w151 -> [w160 _]
            tunnel: w150 -> [w159 w168]
            tunnel: w146 -> [w157 w167]
            tunnel: [w156 w165] -> w145
            tunnel: w144 -> [w155 w170]
            tunnel: w140 -> [_ w166]
            tunnel: w138 -> [w153 w164]
            frame False {
              # "Current ROI"
              n50 = call "AlliGator Get Current ROI Name.vi"() -> ("Current ROI Name"=w154:string)  [unwired: 9 in]
              n51 = call "Image Display Get ROI Characteristics.vi"("ROI Characteristics Selection"=w153, "Error In"=w155, "ROI Mask refnum"=w157, "Image refnum"=w159, "Image Control Refnum"=w160) -> ("Error Out"=w163:errorcluster, "ROI"=w161:T67, "ROI Characteristics String"=w158:string)  [unwired: 3 in, 1 out]
              n52 = call "Get ROI Statistics String.vi"("error in (no error)"=w163, "ROI"=w161, "ROI Name (\"\")"=w154, "ROI Statistics String"=w158) -> ("error out"=w162:errorcluster, "Message"=w156:string)  [unwired: 6 in]
            }
            frame True {
              # "All ROIs"
              n53 = call "AlliGator Compute & Plot All ROIs Characteristics.vi"("ROI Statistics Selection"=w164, "Lifetime Graph"=w166, "error in (no error)"=w170, "ROI Mask Refnum"=w167, "Source Image Refnum"=w168) -> ("error out"=w169:errorcluster, "ROI Statistics String"=w165:string)  [unwired: 5 in]
            }
          }
          n54 = call "Hide Animated Busy Icon with Message.vi"("Already active? (F)"=w136, "Error In"=w152, "Target VI reference"=w137) -> ("Error Out"=w142:errorcluster)  [unwired: 8 in]
        }
      }
    }
    frame "Image:Convert ROI to Mask Image" {
      # "Image:Convert ROI to Mask Image"
      n55 = call-poly "Variant to Data.vi"("Variant"=w179) -> ("Value"=w171:bool)  [unwired: 8 in]
      n56 = call "Show Animated Busy Icon with Message.vi"("Already active? (F)"=w172, "Message"=w175, "Error In"=w177, "Target VI Refnum"=w173) -> ("Error Out"=w176:errorcluster)  [unwired: 7 in]
      n57 = call "AlliGator ROIs to Mask Image.vi"("error in"=w176, "All ROIs?"=w171, "Data Value Reference in"=w181) -> ("error out"=w182:errorcluster, "Message"=w178:string, "Data Value Reference out"=w180:refnum<data-value>)  [unwired: 6 in]
      n58 = call "Hide Animated Busy Icon with Message.vi"("Already active? (F)"=w172, "Error In"=w182, "Target VI reference"=w173) -> ("Error Out"=w174:errorcluster)  [unwired: 8 in]
    }
    frame "Image:Copy Image to Clipboard" {
      # "\"Copy Image to Clipboard\""
      n59 = Variant To Data(type=T19 {"CtlRef"=refnum, "Image to Clipboard Options"={"Include Overlay (T)"=FALSE, "Image Only (T)"=FALSE}} ("output cluster"), Variant=w192) -> (data=w191:T19, error out=w190:errorcluster)  [unwired: 1 in]
      n60 = Unbundle(w191) -> ("CtlRef"=w188:refnum<vi>, "Image to Clipboard Options"=w187:T18)
      n61 = call "Image Display Copy Image to Clipboard.vi"("Error In"=w190, "Image to Clipboard Options"=w187, "Display Image Control Refnum"=w188) -> ("Error Out"=w185:errorcluster)  [unwired: 8 in]
    }
    frame "Image:Create Complementary ROI" {
      # "Create Complementary ROI"
      n62 = Unbundle By Name(w207) -> ("Registered Events Ctrl Refnums.Source Image Display"=w209:refnum<vi>)
      n63 = property on="Property Node" class="ImageControl"(reference=w209) -> (error out=w199:errorcluster, "Label.Text"=w195:string, "ROI"=w196:T67, "Value"=w200:variant)  [unwired: 1 in, 1 out]
      n64 = Variant To Data(error in=w199, Variant=w200) -> (data=w197:T24, error out=w198:errorcluster)  [unwired: 1 in]
      n65 = call "Show Animated Busy Icon with Message.vi"("Already active? (F)"=w194, "Message"=w208, "Error In"=w198, "Target VI Refnum"=w204) -> ("Error Out"=w203:errorcluster)  [unwired: 7 in]
      n66 = call "AlliGator Create Complementary ROI.vi"("Image Label"=w195, "Error In"=w203, "ROI"=w196, "Image"=w197) -> ("Error Out"=w205:errorcluster, "Message"=w201:string)  [unwired: 6 in]
      n67 = call "Hide Animated Busy Icon with Message.vi"("Already active? (F)"=w194, "Error In"=w205, "Target VI reference"=w204) -> ("Error Out"=w206:errorcluster)  [unwired: 8 in]
    }
    frame "Image:Create Contour ROI" {
      # "Create Contour ROI (deprecated)"
      n68 = Unbundle By Name(w228) -> ("Registered Events Ctrl Refnums.Source Image Display"=w230:refnum<vi>)
      n69 = call "AlliGator IV ROI Mask.vi"("Get (F)/ Set (T)"=FALSE, "AlliGator IV DVR in"=w223) -> ("error out"=w211:errorcluster, "ROI Mask Image"=w212:T24, "AlliGator IV DVR out"=w214:refnum<data-value>)  [unwired: 7 in]
      n70 = property on="Property Node" class="ImageControl"(reference=w230, error in=w211) -> (error out=w220:errorcluster, "ROI"=w217:T67, "Value"=w221:variant, "Label.Text"=w215:string)  [unwired: 1 out]
      n71 = Variant To Data(error in=w220, Variant=w221) -> (data=w218:T24, error out=w219:errorcluster)  [unwired: 1 in]
      n72 = call "Show Animated Busy Icon with Message.vi"("Already active? (F)"=w216, "Message"=w229, "Error In"=w219, "Target VI Refnum"=w225) -> ("Error Out"=w224:errorcluster)  [unwired: 7 in]
      n73 = call "AlliGator Create Source Image Contour ROI.vi"("Image Label"=w215, "ROI Mask"=w212, "Error In"=w224, "ROI"=w217, "Image"=w218) -> ("Error Out"=w226:errorcluster, "Message"=w222:string)  [unwired: 5 in]
      n74 = call "Hide Animated Busy Icon with Message.vi"("Already active? (F)"=w216, "Error In"=w226, "Target VI reference"=w225) -> ("Error Out"=w227:errorcluster)  [unwired: 8 in]
    }
    frame "Image:Create ROI Grid" {
      # "\"Create ROI Grid\""
      n75 = Unbundle By Name(w235) -> ("Registered Events Ctrl Refnums.Source Image Display"=w237:refnum<vi>)
      n76 = property on="Property Node" class="ImageControl"(reference=w237) -> (error out=w242:errorcluster, "ROI"=w243:T67)  [unwired: 1 in, 1 out]
      n77 = call "Show Animated Busy Icon with Message and Abort Button.vi"("Already active? (F)"=w238, "Message"=w236, "Target VI reference"=w234, "Error In"=w242) -> ("Error Out"=w240:errorcluster)  [unwired: 15 in]
      n78 = call "AlliGator Create Source Image ROI Grid.vi"("Error In"=w240, "ROI"=w243) -> ("Error Out"=w241:errorcluster, "Message"=w232:string)  [unwired: 8 in]
      n79 = call "Hide Animated Busy Icon with Message and Abort Button.vi"("Already active? (F)"=w238, "Target VI reference"=w234, "Error In"=w241) -> ("Error Out"=w239:errorcluster)  [unwired: 16 in]
    }
    frame "Image:Create ROI(s) from Pixels with Intensity above Min_Scriptable" {
      w247 = TRUE  # Sum
      # "\"Create ROI(s) from Pixels with Intensity above Min\""
      n80 = call "AlliGator IV Selected Max or Sum Image.vi"("Sum (T)/ Max (F)"=w247, "AlliGator IV DVR in"=w249) -> ("Error Out"=w248:errorcluster, "Selected Gate Image (Sum/Max)"=w251:T24, "Current Folder"=w266:path, "AlliGator IV DVR out"=w250:refnum<data-value>)  [unwired: 6 in]
      n81 = call "Show Animated Busy Icon with Message.vi"("Already active? (F)"=w245, "Message"=w263, "Error In"=w248, "Target VI Refnum"=w252) -> ("Error Out"=w262:errorcluster)  [unwired: 7 in]
      n82 = call "AlliGator Settings Storage.vi"("Get(F)/Set"=FALSE, "AlliGator Settings List"=AlliGator_Settings_List."Source Image:Intensity Threshold", "Error In"=w262) -> ("Error Out"=w256:errorcluster, "Variant Data out"=w259:variant)  [unwired: 7 in]
      n83 = call-poly "Variant to Data.vi"("Variant"=w259) -> ("Value"=w254:dbl)  [unwired: 8 in]
      n84 = call "Threshold Max Image to ROIs.vi"("Error In"=w256, "Threshold"=w254, "Image Refnum in"=w251) -> ("Error Out"=w257:errorcluster, "ROIs"=w258:T22[])  [unwired: 7 in]
      n85 = Format Into String(format string="Computing ROIs based on Min Intensity %#g:\n", w254) -> (resulting string=w253:string)  [unwired: 2 in, 1 out]
      n86 = call "AlliGator Add Multiple Source Image ROIs.vi"("Header message"=w253, "Error In"=w257, "ROIs"=w258, "ROI Mask Image Path"=w266) -> ("Error Out"=w265:errorcluster, "Message"=w246:string)  [unwired: 6 in]
      n87 = call "Hide Animated Busy Icon with Message.vi"("Already active? (F)"=w245, "Error In"=w265, "Target VI reference"=w252) -> ("Error Out"=w264:errorcluster)  [unwired: 8 in]
    }
    frame "Image:Create ROI(s) from Pixels with Peak above Min_Scriptable" {
      w270 = FALSE  # Max
      # "\"Create ROI from Pixels with Peak above Min\""
      n88 = call "AlliGator IV Selected Max or Sum Image.vi"("Sum (T)/ Max (F)"=w270, "AlliGator IV DVR in"=w274) -> ("Selected Gate Image (Sum/Max)"=w271:T24, "Current Folder"=w273:path, "AlliGator IV DVR out"=w272:refnum<data-value>)  [unwired: 6 in, 1 out]
      n89 = call "Show Animated Busy Icon with Message.vi"("Already active? (F)"=w268, "Message"=w285, "Target VI Refnum"=w275) -> ("Error Out"=w288:errorcluster)  [unwired: 8 in]
      n90 = call "AlliGator Settings Storage.vi"("Get(F)/Set"=FALSE, "AlliGator Settings List"=AlliGator_Settings_List."Source Image:Peak Threshold", "Error In"=w288) -> ("Error Out"=w279:errorcluster, "Variant Data out"=w282:variant)  [unwired: 7 in]
      n91 = call-poly "Variant to Data.vi"("Variant"=w282) -> ("Value"=w277:dbl)  [unwired: 8 in]
      n92 = call "Threshold Max Image to ROIs.vi"("Error In"=w279, "Threshold"=w277, "Image Refnum in"=w271) -> ("Error Out"=w280:errorcluster, "ROIs"=w281:T22[])  [unwired: 7 in]
      n93 = Format Into String(format string="Computing ROIs based on Min Peak Value %#g:\n", w277) -> (resulting string=w276:string)  [unwired: 2 in, 1 out]
      n94 = call "AlliGator Add Multiple Source Image ROIs.vi"("Header message"=w276, "Error In"=w280, "ROIs"=w281, "ROI Mask Image Path"=w273) -> ("Error Out"=w287:errorcluster, "Message"=w269:string)  [unwired: 6 in]
      n95 = call "Hide Animated Busy Icon with Message.vi"("Already active? (F)"=w268, "Error In"=w287, "Target VI reference"=w275) -> ("Error Out"=w286:errorcluster)  [unwired: 8 in]
    }
    frame "Image:Delete All ROIs" {
      # "\"Image:Delete All ROIs\""
      n96 = Bundle By Name(cluster=T4 {"AlliGator Q Event"=enum."Image:Source Image ROI Storage", "Data"=variant} ("Alligator Atomic Action"), "Data"=AlliGator_ROI_Manager_Actions."Delete All ROIs" ("Action")) -> (w293:T4)
      n97 = call-poly "AlliGator Add Action(s) to Stack.vi"("Elements Order in Action Stack (Default: 2 BEFORE 1)"=Alligator_Elements_Order_in_Action_Stack."Enqueue 2 BEFORE 1", "Error In"=w291, "Alligator Atomic Action"=w293, "Alligator Queue Element 1"=w299) -> ("Error Out"=w290:errorcluster, "Alligator Queue Element 1 (+ 2)"=w296:T4[])  [unwired: 6 in]
    }
    frame "Image:Delete All Unselected ROIs" {
      # "\"Image:Delete All Unselected ROIs\""
      n98 = Bundle By Name(cluster=T4 {"AlliGator Q Event"=enum."Image:Source Image ROI Storage", "Data"=variant} ("Alligator Atomic Action"), "Data"=AlliGator_ROI_Manager_Actions."Delete All Unselected ROIs" ("Action")) -> (w303:T4)
      n99 = call-poly "AlliGator Add Action(s) to Stack.vi"("Elements Order in Action Stack (Default: 2 BEFORE 1)"=Alligator_Elements_Order_in_Action_Stack."Enqueue 2 BEFORE 1", "Error In"=w301, "Alligator Atomic Action"=w303, "Alligator Queue Element 1"=w309) -> ("Error Out"=w300:errorcluster, "Alligator Queue Element 1 (+ 2)"=w306:T4[])  [unwired: 6 in]
    }
    frame "Image:Delete Existing ROIs Option" {
      # "\"Image:Delete Existing ROIs Option\""
      n100 = call "AlliGator skippable_Delete Existing ROIs Dialog Window.vi"("Error In"=w311) -> ("Error Out"=w314:errorcluster, "Delete"=w313:bool)  [unwired: 9 in]
      n101 = case shown="True" w313 {
        tunnel: w314 -> [w318 w323]
        tunnel: [w318 w321] -> w312
        tunnel: [_ w320] -> w310
        frame False {
        }
        frame True {
          n102 = call-poly "AlliGator Source Image ROI Storage [PM].vi"("Error In"=w323, "Current ROI Descriptor"=T22 {"Global Rectangle"=[], "Contours"=[]}, "Action"=AlliGator_ROI_Manager_Actions."Delete All ROIs") -> ("Error Out"=w321:errorcluster, "Message"=w320:string)  [unwired: 2 in, 5 out]
        }
      }
    }
    frame "Image:Delete ROI" {
      # "\"Image:Delete ROI\""
      n103 = Bundle By Name(cluster=T4 {"AlliGator Q Event"=enum."Image:Source Image ROI Storage", "Data"=variant} ("Alligator Atomic Action"), "Data"=AlliGator_ROI_Manager_Actions."Delete Current ROI" ("Action")) -> (w327:T4)
      n104 = call-poly "AlliGator Add Action(s) to Stack.vi"("Elements Order in Action Stack (Default: 2 BEFORE 1)"=Alligator_Elements_Order_in_Action_Stack."Enqueue 2 BEFORE 1", "Error In"=w325, "Alligator Atomic Action"=w327, "Alligator Queue Element 1"=w333) -> ("Error Out"=w324:errorcluster, "Alligator Queue Element 1 (+ 2)"=w330:T4[])  [unwired: 6 in]
    }
    frame "Image:Delete ROI(s) based on ROI Characteristics" {
      n105 = call "AlliGator Get Selected Image to Display.vi"("Error In"=w341, "AlliGator IV DVR in"=w345) -> ("Error Out"=w346:errorcluster, "Image out"=w342:T24, "AlliGator IV DVR out"=w344:refnum<data-value>, "ROI Mask"=w338:T24)  [unwired: 4 in, 2 out]
      n106 = call "Show Animated Busy Icon with Message.vi"("Already active? (F)"=w334, "Message"=w339, "Error In"=w346, "Target VI Refnum"=w335) -> ("Error Out"=w343:errorcluster)  [unwired: 7 in]
      n107 = case shown="No Error" w343 {
        selector: w343 -> [w352 w353]
        tunnel: w342 -> [w351 _]
        tunnel: w338 -> [w350 _]
        tunnel: [w349 _] -> w340
        tunnel: [w348 w353] -> w337
        frame No Error {
          n108 = call "AlliGator Reject Source Image ROIs based on Characteristics.vi"("error in (no error)"=w352, "ROI Mask Refnum"=w350, "Source Image Refnum"=w351) -> ("error out"=w348:errorcluster, "ROI Characteristics String"=w349:string)  [unwired: 7 in]
        }
        frame Error {
        }
      }
      n109 = call "Hide Animated Busy Icon with Message.vi"("Already active? (F)"=w334, "Error In"=w337, "Target VI reference"=w335) -> ("Error Out"=w336:errorcluster)  [unwired: 8 in]
    }
    frame "Image:Export ROI Description to Notebook" {
      # "\"Export ROI Description to Notebook\""
      n110 = Variant To Data(type=T23 {"Image Control Label"="", "ROI Descriptor"={"Global Rectangle"=[], "Contours"=[]}} ("cluster"), Variant=w369) -> (data=w356:T23, error out=w358:errorcluster)  [unwired: 1 in]
      n111 = case shown="Error .." w358 {
        selector: w358 -> [w371 _]
        tunnel: [w373 w376] -> w365
        tunnel: w356 -> [w372 w377]
        tunnel: w357 -> [_ w380]
        tunnel: [w372 w378] -> w355
        tunnel: [w371 w374] -> w354
        frame No Error {
          n112 = Unbundle By Name(w372) -> ("ROI Descriptor"=w373:T22)
        }
        frame Error {
          n113 = Unbundle By Name(w380) -> ("Registered Events Ctrl Refnums.Source Image Display"=w379:refnum<vi>)
          n114 = property class="ImageControl"(reference=w379) -> (error out=w374:errorcluster, "ROI"=w376:T67)  [unwired: 1 in, 1 out]
          n115 = Bundle By Name(cluster=w377, "ROI Descriptor"=w376, "Image Control Label"="Source Image") -> (w378:T23)
        }
      }
      n116 = call "Get ROI Area.vi"("Error In"=w354, "ROI Descriptor"=w365) -> ("Error Out"=w364:errorcluster, "Number of Pixels"=w363:u32)  [unwired: 8 in]
      n117 = call "AlliGator Find ROI Name.vi"("Error In"=w364, "ROI Descriptor"=w355) -> ("Error Out"=w367:errorcluster, "Image Control ROI Description"=w366:T68)  [unwired: 7 in, 1 out]
      n118 = call "AlliGator Format ROI Description for Notebook.vi"("error in (no error)"=w367, "# Pixels"=w363, "ROI Descriptor"=w366) -> ("error out"=w361:errorcluster, "Message"=w359:string)  [unwired: 7 in]
    }
    frame "Image:Identify ROIs in Mask Image" {
      # "\"Identify ROIs in Mask Image\""
      n119 = call-poly "Variant to Data.vi"("Variant"=w389) -> ("String"=w388:string)  [unwired: 8 in]
      n120 = call "Show Animated Busy Icon with Message.vi"("Already active? (F)"=w381, "Message"=w384, "Error In"=w386, "Target VI Refnum"=w382) -> ("Error Out"=w385:errorcluster)  [unwired: 7 in]
      n121 = call "AlliGator Mask Image to ROIs.vi"("error in"=w385, "Mask Image Name (Default: none)"=w388, "Data Value Reference in"=w391) -> ("error out"=w392:errorcluster, "Message"=w387:string, "Data Value Reference out"=w390:refnum<data-value>)  [unwired: 6 in]
      n122 = call "Hide Animated Busy Icon with Message.vi"("Already active? (F)"=w381, "Error In"=w392, "Target VI reference"=w382) -> ("Error Out"=w383:errorcluster)  [unwired: 8 in]
    }
    frame "Image:Image Contrast" {
      w415 = -1074396120  # Not an image
      # "\"Image Contrast\""
      n123 = Variant To Data(type=T24 refnum ("Image out"), Variant=w398) -> (data=w396:T24, error out=w397:errorcluster)  [unwired: 1 in]
      n124 = call "Show Animated Busy Icon with Message.vi"("Already active? (F)"=w403, "Message"=w409, "Target VI Refnum"=w410) -> ("Error Out"=w419:errorcluster)  [unwired: 8 in]
      n125 = Unbundle By Name(w411) -> ("Dataset Control References.Image Color Scale"=w412:refnum<vi>, "Registered Events Ctrl Refnums.Source Image Display"=w401:refnum<vi>, "Image Histogram Ctrl Refnums.Image Histogram"=w400:refnum<vi>)
      n126 = call "AlliGator Get Selected Image to Display.vi"("Error In"=w419, "AlliGator IV DVR in"=w408) -> ("Error Out"=w406:errorcluster, 1:"Displayed Image"=w413:T24, "Image out"=w395:T24, "AlliGator IV DVR out"=w407:refnum<data-value>, 4:"Displayed Image"=w405:T36)  [unwired: 4 in, 1 out]
      n127 = call "Alligator Variables Storage.vi"("Get(F)/Set"=FALSE, "AlliGator Variable"=AlliGator_Variables_List."X_Source Image Palette Information" ("Alligator Variable"), "Error In"=w406) -> ("Error Out"=w418:errorcluster, "Data out"=w424:variant)  [unwired: 6 in, 1 out]
      n128 = Select(t=w395, s=w397, f=w396) -> (s? t:f=w394:T24)
      n129 = Variant To Data(error in=w418, type=T16 {"Palette Name [# Colors,int?,inv?]"="", "Palette Type"=0, "Palette Colors"=[], "Interpolate?"=FALSE} ("Image Display Palette Information"), Variant=w424) -> (data=w421:T16, error out=w416:errorcluster)
      n130 = call "AlliGator Set Image Display Range.vi"("Display Image Control Refnum"=w401, "Image Histogram"=w400, "Error In"=w406, "Displayed Image?"=w405, "Displayed Image"=w413, "Image to Display"=w394) -> ("Error Out"=w425:errorcluster, "Palette Display Range"=w422:cluster{"Min Value":dbl, "Max Value":dbl}, "Image Display Range"=w402:cluster{"Min Value":dbl, "Max Value":dbl})  [unwired: 2 in, 1 out]
      n131 = Merge Errors(w425, w416) -> (w417:errorcluster)
      n132 = case shown="\"Single Gate\", Default" w405 {
        tunnel: w417 -> [w439 w440]
        tunnel: w422 -> [w431 _]
        tunnel: w421 -> [w436 _]
        tunnel: w412 -> [w438 _]
        tunnel: w401 -> [w437 _]
        tunnel: [w435 w440] -> w404
        tunnel: w402 -> [w432 _]
        frame "Single Gate", Default {
          n133 = property on="Property Node" class="ColRmp (strict)"(reference=w438) -> (reference out=w433:refnum<vi>, "Scale.High Color"=w429:u32, "Scale.Low Color"=w430:u32)  [unwired: 1 in, 1 out]
          n134 = call "Image Display Set Color Palette.vi"("Image High Color"=w429, "Image Low Color"=w430, "Error In"=w439, "Image Display Range"=w432, "Image Display Palette Information"=w436, "Display Image Control Refnum"=w437) -> ("Error Out"=w434:errorcluster)  [unwired: 5 in]
          n135 = call "Set Color Ramp Palette v3.vi"("Image High Color"=w429, "Image Low Color"=w430, "error in (no error)"=w434, "Image Display Range"=w431, "Image Display Palette Information"=w436, "ColorRamp in"=w433) -> ("Error Out"=w435:errorcluster)  [unwired: 3 in, 2 out]
        }
        frame "Mask Image" {
        }
      }
      n136 = call "Hide Animated Busy Icon with Message.vi"("Already active? (F)"=w403, "Error In"=w404, "Target VI reference"=w410) -> ("Error Out"=w414:errorcluster)  [unwired: 8 in]
      n137 = call <vilib>:"Clear Errors.vi"("error in (no error)"=w414, "specific error code to clear (0: all)"=w415) -> ("error out"=w427:errorcluster)  [unwired: 4 in, 1 out]
    }
    frame "Image:Image Histogram Cursor Move" {
      n138 = Bundle By Name(cluster=T4 {"AlliGator Q Event"=enum."Image:Set Image Histogram Cursor Move Flag", "Data"=variant} ("element"), "Data"=FALSE) -> (w442:T4)
      n139 = Build Array (concatenate)(T4[] [{"AlliGator Q Event"=enum."Image:Image Histogram", "Data"=variant}, {"AlliGator Q Event"=enum."Image:Image Contrast", "Data"=variant}] ("element"), w442) -> (w444:T4[])
      n140 = call-poly "AlliGator Add Action(s) to Stack.vi"("Elements Order in Action Stack (Default: 2 BEFORE 1)"=Alligator_Elements_Order_in_Action_Stack."Enqueue 2 BEFORE 1", "Alligator Queue Element 2"=w444, "Alligator Queue Element 1"=w448) -> ("Alligator Queue Element 1 (+ 2)"=w446:T4[])  [unwired: 7 in, 1 out]
    }
    frame "Image:Image Histogram" {
      # "\"Image Histogram\""
      n141 = Unbundle By Name(w457) -> ("Image Histogram Ctrl Refnums.Image Histogram Active"=w458:refnum<vi>)
      n142 = property on="Property Node" class="Bool (strict)"(reference=w458) -> ("Value"=w456:bool)  [unwired: 1 in, 2 out]
      n143 = case shown="True" w456 {
        tunnel: w461 -> [_ w483]
        tunnel: w460 -> [_ w479]
        tunnel: [_ w485] -> w459
        tunnel: w457 -> [_ w484]
        tunnel: w455 -> [_ w480]
        tunnel: w454 -> [w463 w482]
        tunnel: [w463 w481] -> w453
        tunnel: w452 -> [_ w468]
        frame False {
        }
        frame True {
          n144 = Variant To Data(type=T24 refnum ("Image out"), Variant=w468) -> (data=w465:T24, error out=w466:errorcluster)  [unwired: 1 in]
          n145 = call "Show Animated Busy Icon with Message.vi"("Already active? (F)"=w479, "Message"=w480, "Target VI Refnum"=w483) -> ("Error Out"=w478:errorcluster)  [unwired: 8 in]
          n146 = Unbundle By Name(w484) -> ("Dataset Control References.Gate Image Slide"=w469:refnum<vi>, "Image Histogram Ctrl Refnums"=w476:T12, "Dataset Control References.Displayed Image"=w464:refnum<vi>)
          n147 = case shown="Error .." w466 {
            tunnel: w482 -> [w490 w496]
            tunnel: [w490 w495] -> w481
            tunnel: w478 -> [w488 w494]
            tunnel: [w489 w493] -> w475
            tunnel: [w488 w492] -> w473
            tunnel: [w486 w491] -> w472
            tunnel: w465 -> [w489 _]
            tunnel: w464 -> [w487 _]
            frame No Error {
              n148 = property class="Enum (strict)"(reference=w487) -> ("Value"=w486:T36)  [unwired: 1 in, 2 out]
            }
            frame Error {
              n149 = call "AlliGator Get Selected Image to Display.vi"("Error In"=w494, "AlliGator IV DVR in"=w496) -> ("Error Out"=w492:errorcluster, "Image out"=w493:T24, "AlliGator IV DVR out"=w495:refnum<data-value>, "Displayed Image"=w491:T36)  [unwired: 4 in, 2 out]
            }
          }
          n150 = case shown="\"Sum of All Gates\", Default" w472 {
            selector: w472 -> [w499 w502]
            tunnel: [TRUE ("Visible") _] -> w474
            tunnel: [w499 w502] -> w471
            tunnel: w469 -> [w498 _]
            tunnel: [w497 u16 0 ("Value")] -> w470
            frame "Single Gate" {
              n151 = property on="Property Node" class="Slide (strict)"(reference=w498) -> ("Value"=w497:u16)  [unwired: 1 in, 2 out]
            }
            frame "Sum of All Gates", Default {
            }
          }
          n152 = property on="Property Node" class="Slide (strict)"(reference=w469, "Visible"=w474) -> ()  [unwired: 1 in, 2 out]
          n153 = call "AlliGator Single Image Histogram.vi"("Gate Slider"=w470, "Error In"=w473, "Displayed Image"=w471, "Image Histogram Ctrl Refnums"=w476, "Image in"=w475) -> ("Error Out"=w477:errorcluster)  [unwired: 3 in, 3 out]
          n154 = call "Hide Animated Busy Icon with Message.vi"("Already active? (F)"=w479, "Error In"=w477, "Target VI reference"=w483) -> ("Error Out"=w485:errorcluster)  [unwired: 8 in]
        }
      }
    }
    frame "Image:Load ROI" {
      # "\"Load ROI\""
      n155 = Variant To Data(error in=w504, type=refnum<vi> refnum ("CtlRef"), Variant=w516) -> (data=w514:refnum<vi>, error out=w513:errorcluster)
      n156 = call "Show Animated Busy Icon with Message.vi"("Already active? (F)"=w505, "Message"=w503, "Error In"=w513, "Target VI Refnum"=w508) -> ("Error Out"=w511:errorcluster)  [unwired: 7 in]
      n157 = call "AlliGator Load ROI v3.vi"("Error In"=w511, "Dialog (T)"=TRUE, "Source Image Refnum"=w514) -> ("Error Out"=w512:errorcluster, "Message"=w506:string)  [unwired: 2 in, 5 out]
      n158 = call "Hide Animated Busy Icon with Message.vi"("Already active? (F)"=w505, "Error In"=w512, "Target VI reference"=w508) -> ("Error Out"=w510:errorcluster)  [unwired: 8 in]
    }
    frame "Image:Merge All ROIs" {
      # "\"Image:Merge All ROIs\""
      n159 = Bundle By Name(cluster=T4 {"AlliGator Q Event"=enum."Image:Source Image ROI Storage", "Data"=variant} ("Alligator Atomic Action"), "Data"=AlliGator_ROI_Manager_Actions."Merge All ROIs" ("Action")) -> (w521:T4)
      n160 = call-poly "AlliGator Add Action(s) to Stack.vi"("Elements Order in Action Stack (Default: 2 BEFORE 1)"=Alligator_Elements_Order_in_Action_Stack."Enqueue 2 BEFORE 1", "Error In"=w519, "Alligator Atomic Action"=w521, "Alligator Queue Element 1"=w527) -> ("Error Out"=w518:errorcluster, "Alligator Queue Element 1 (+ 2)"=w524:T4[])  [unwired: 6 in]
    }
    frame "Image:Mouse Move" {
      # "\"Image:Mouse Move\""
      n161 = Variant To Data(error in=w528, Variant=w532) -> (data=w531:T69, error out=w530:errorcluster)  [unwired: 1 in]
      n162 = call "AlliGator Source Image Mouse Move Event.vi"("error in"=w530, "Image User Event Data"=w531, "AlliGator Events in"=w534) -> ("error out"=w529:errorcluster, "AlliGator Events out"=w533:T4[])  [unwired: 7 in]
    }
    frame "Image:Mouse Up" {
      # "\"Image:Mouse Up\""
      n163 = Unbundle By Name(w539) -> ("Registered Events Ctrl Refnums.Source Image Display"=w538:refnum<vi>, "Dataset Control References"=w537:T10)
      n164 = Variant To Data(error in=w545, Variant=w546) -> (data=w540:T71, error out=w541:errorcluster)  [unwired: 1 in]
      n165 = call "AlliGator Source Image Mouse Up Event.vi"("Dataset Ctrl Refnums"=w537, "error in (no error)"=w541, "Phasor Plot Mouse Up Event Data"=w540, "Image Control Refnum"=w538, "AlliGator Actions in"=w544) -> ("error out"=w542:errorcluster, "AlliGator Actions out"=w543:T4[])  [unwired: 5 in]
    }
    frame "Image:Overlay ROI Median" {
      # "\"Image:Overlay ROI Median\""
      n166 = call "AlliGator Overlay ROI Median.vi"("AlliGator Ctrl Refnums"=w551, "error in (no error)"=w549, "AlliGator IV DVR in"=w553) -> ("error out"=w550:errorcluster, "AlliGator IV DVR out"=w552:refnum<data-value>)  [unwired: 7 in]
    }
    frame "Image:Paste ROI Definition" {
      # "\"Paste ROI Definition\""
      n167 = Unbundle By Name(w560) -> ("Registered Events Ctrl Refnums.Source Image Display"=w559:refnum<vi>)
      n168 = invoke on="Invoke Node" class="App" method="Clipboard.Read"() -> (error out=w566:errorcluster, "Read Clipbrd"=w567:string)  [unwired: 3 in, 1 out]
      n169 = call "ROI Description to ROI.vi"("error in (no error)"=w566, "ROI Description"=w567) -> ("error out"=w565:errorcluster, "Current ROI Descriptor(s)"=w564:T22)  [unwired: 8 in]
      n170 = disable-structure "Diagram Disable Structure" shown="Enabled" {
        disable-tunnel: w565 -> [w575 w576]
        disable-tunnel: w564 -> [w574 w577]
        disable-tunnel: [w572 w576] -> w563
        disable-tunnel: [w571 w577] -> w562
        disable-tunnel: [w570 _] -> w556
        frame Disabled {
          n171 = call-poly "AlliGator Source Image ROI Storage [PM].vi"("Error In"=w575, "Current ROI Descriptor"=w574, "Action"=AlliGator_ROI_Manager_Actions."Store New ROI" ("Enum")) -> ("Error Out"=w572:errorcluster, "Current ROI Descriptor"=w571:T22, "Message"=w570:string)  [unwired: 2 in, 4 out]
        }
        frame Enabled {
        }
      }
      n172 = call "Image Display Get-Set ROI.vi"("Get(F)/Set"=TRUE ("Get(F)/Set(T)"), "Error In"=w563, "ROI Descriptor in"=w562, "Image Display Refnum"=w559) -> ("Error Out"=w561:errorcluster)  [unwired: 3 in, 4 out]
    }
    frame "Image:Python Function Source Image Event" {
      # "\"Python Function Source Image Event\""
      n173 = Variant To Data(Variant=w594) -> (data=w593:T76, error out=w592:errorcluster)  [unwired: 2 in]
      n174 = call "Show Animated Busy Icon with Message.vi"("Already active? (F)"=w578, "Message"=w591, "Error In"=w592, "Target VI Refnum"=w590) -> ("Error Out"=w580:errorcluster)  [unwired: 7 in]
      n175 = call "AlliGator Image Python Function Handler Core.vi"("error in (no error)"=w580, "Data Value Reference in"=w583, "Image Event"=w593) -> ("error out"=w581:errorcluster, "Message"=w579:string, "Data Value Reference out"=w582:refnum<data-value>, "Alligator Atomic Action"=w584:T4[])  [unwired: 5 in]
      n176 = call "Hide Animated Busy Icon with Message.vi"("Already active? (F)"=w578, "Error In"=w581, "Target VI reference"=w590) -> ("Error Out"=w587:errorcluster)  [unwired: 8 in]
      n177 = call-poly "AlliGator Add Action(s) to Stack.vi"("Elements Order in Action Stack (Default: 2 BEFORE 1)"=Alligator_Elements_Order_in_Action_Stack."Enqueue 2 BEFORE 1", "Error In"=w587, "Alligator Queue Element 2"=w584, "Alligator Queue Element 1"=w589) -> ("Error Out"=w585:errorcluster, "Alligator Queue Element 1 (+ 2)"=w588:T4[])  [unwired: 6 in]
    }
    frame "Image:ROI to Individual Pixel ROIs" {
      w595 = FALSE ("Get (F)/ Set (T)")
      w600 = "Abort ROI Creation" ("Abort Button Name (Abort)")
      # "\"ROI to Individual Pixel ROIs\""
      n178 = Unbundle By Name(w613) -> ("Registered Events Ctrl Refnums.Source Image Display"=w615:refnum<vi>, "Other AlliGator Ctrl Refnums.Abort ROI Creation"=w607:refnum<vi>)
      n179 = call "AlliGator IV Type of Displayed Image.vi"("Get (F)/ Set (T)"=w595, "AlliGator IV DVR in"=w605) -> ("error out"=w597:errorcluster, "Type of Displayed Image"=w596:T36, "AlliGator IV DVR out"=w598:refnum<data-value>)  [unwired: 7 in]
      n180 = case shown="\"Mask Image\"" w596 {
        tunnel: [w626 w629 w635] -> w604
        tunnel: [w625 w630 w636] -> w603
        tunnel: [w624 w628 w634] -> w602
        tunnel: w598 -> [w622 w632 w638]
        tunnel: w597 -> [w621 w631 w637]
        tunnel: w595 -> [_ w627 w633]
        frame "Single Gate", Default {
          n181 = call "AlliGator IV Selected Max or Sum Image.vi"("Error In"=w621, "Sum (T)/ Max (F)"=FALSE, "AlliGator IV DVR in"=w622) -> ("Error Out"=w624:errorcluster, "Selected Gate Image (Sum/Max)"=w626:T24, "AlliGator IV DVR out"=w625:refnum<data-value>)  [unwired: 5 in, 1 out]
        }
        frame "White Ligth Image" {
          n182 = call "AlliGator IV White Light Image.vi"("Get (F)/ Set (T)"=w627, "error in (no error)"=w631, "AlliGator IV DVR in"=w632) -> ("error out"=w628:errorcluster, "White Light Image"=w629:T24, "AlliGator IV DVR out"=w630:refnum<data-value>)  [unwired: 6 in]
        }
        frame "Mask Image" {
          n183 = call "AlliGator IV Mask Image.vi"("Get (F)/ Set (T)"=w633, "error in (no error)"=w637, "AlliGator IV DVR in"=w638) -> ("error out"=w634:errorcluster, "Mask Image"=w635:T24, "AlliGator IV DVR out"=w636:refnum<data-value>)  [unwired: 6 in]
        }
      }
      n184 = call-poly "Variant to Data.vi"("Variant"=w610) -> ("Value"=w609:i32)  [unwired: 8 in]
      n185 = property on="Property Node" class="ImageControl"(reference=w615, error in=w602) -> (error out=w619:errorcluster, "ROI"=w618:T67)  [unwired: 1 out]
      n186 = call "Show Animated Busy Icon with Message and Abort Button.vi"("Already active? (F)"=w599, "Message"=w614, "Target VI reference"=w608, "Error In"=w619, "Abort Button Name (Abort)"=w600) -> ("Error Out"=w606:errorcluster)  [unwired: 14 in]
      n187 = call "IMAQ GetImageInfo"("Image"=w604) -> ("Y Resolution"=w616:i32, "X Resolution"=w617:i32)  [unwired: 3 in, 6 out]
      n188 = call "AlliGator Create Individual Pixel ROIs from ROI.vi"("Y Resolution"=w616, "X Resolution"=w617, "Error In"=w606, "Abort ROI Creation"=w607, "Selected ROI (-1: use ROI Descriptor)"=w609, "ROI"=w618) -> ("Error Out"=w611:errorcluster, "Message"=w601:string)  [unwired: 4 in]
      n189 = call "Hide Animated Busy Icon with Message and Abort Button.vi"("Already active? (F)"=w599, "Target VI reference"=w608, "Error In"=w611, "Abort Button Name (Abort)"=w600) -> ("Error Out"=w612:errorcluster)  [unwired: 15 in]
    }
    frame "Image:Save Displayed Image with Overlay" {
      # "\"Save Displayed Image with Overlay\""
      n190 = Unbundle By Name(w651) -> ("Registered Events Ctrl Refnums.Source Image Display"=w663:refnum<vi>, "Dataset Control References.Gate Image Slide"=w650:refnum<vi>)
      n191 = call-poly "Variant to Data.vi"("Variant"=w661) -> ("Value"=w657:bool)  [unwired: 8 in]
      n192 = call "AlliGator Get Image File Format.vi"() -> ("error out"=w656:errorcluster, "Transparent Mask Color"=w639:u32, "File Extension (.xxx)"=w653:string, "Image File Format"=w659:T25)  [unwired: 8 in]
      n193 = call "Show Animated Busy Icon with Message.vi"("Already active? (F)"=w640, "Message"=w643, "Error In"=w656, "Target VI Refnum"=w641) -> ("Error Out"=w644:errorcluster)  [unwired: 7 in]
      n194 = call "AlliGator Build Saved Image Path.vi"("Gate Image Slide"=w650, "Error In"=w644, "File Extension"=w653, "AlliGator IV DVR in"=w648) -> ("Error Out"=w655:errorcluster, "appended path"=w654:path, "AlliGator IV DVR out"=w647:refnum<data-value>)  [unwired: 5 in]
      n195 = call "Image File Dialog (Optional).vi"("Dialog?"=w657, "Error In"=w655, "Image File Format in"=w659, "Default file path in"=w654) -> ("Error Out"=w652:errorcluster, "Image File Format out"=w658:T25, "file path out"=w660:path)  [unwired: 5 in]
      n196 = call "Image Display Save Image.vi"("Mask Color (Transparent)"=w639, "error in (no error)"=w652, "Saved Image File Format"=w658, "File Path in"=w660, "Display Image Control Refnum"=w663) -> ("Error Out"=w662:errorcluster, "File Path out"=w649:path)  [unwired: 5 in]
      n197 = call "Hide Animated Busy Icon with Message.vi"("Already active? (F)"=w640, "Error In"=w662, "Target VI reference"=w641) -> ("Error Out"=w642:errorcluster)  [unwired: 8 in]
      n198 = Format Into String(format string="Displayed source Image saved with overlay to %s", error in=w642, w649) -> (resulting string=w646:string, error out=w645:errorcluster)  [unwired: 1 in]
    }
    frame "Image:Save Image as Hot Pixel Mask" {
      # "\"Image:Save Image as Hot Pixel Mask\""
      n199 = in-place "In Place Element Structure" {
        in-place-border: [w708] -> w691
        in-place-border: [w707] -> w690
        in-place-border: [w706] -> w689
        in-place-border: [w704] -> w667
        n200 = in-place-dvr #5 ("Data Value Reference Read / Write Element")(w669) -> (w705:T30, w704:errorcluster)
        n201 = Unbundle By Name(w705) -> ("Single Data Point Path"=w708:path, "[Time-Series Paths]"=w707:path[], "Current Dataset"=w706:i32)
        n202 = in-place-dvr #5 ("Data Value Reference Read / Write Element")() -> (w668:refnum<data-value>)  [unwired: 1 in, 1 out]
      }
      n203 = Unbundle By Name(w695) -> ("Registered Events Ctrl Refnums.Source Image Display"=w681:refnum<vi>)
      n204 = Variant To Data(type=w681, Variant=w682) -> (data=w676:refnum<vi>, error out=w675:errorcluster)  [unwired: 1 in]
      n205 = property on="Property Node" class="ImageControl"(reference=w676, error in=w675) -> (error out=w673:errorcluster, "Value"=w674:variant)  [unwired: 1 out]
      n206 = Variant To Data(error in=w673, Variant=w674) -> (data=w672:T24, error out=w671:errorcluster)  [unwired: 1 in]
      n207 = call "AlliGator Get Destination Folder.vi"("Current Data Set (-1: single)"=w689, "Time-Series Paths"=w690, "Single Data Point Path"=w691) -> ("Data Point Name"=w670:string, "Destination Folder path"=w701:path)  [unwired: 6 in, 1 out]
      n208 = Merge Errors(w671, w667) -> (w680:errorcluster)
      n209 = call "Show Animated Busy Icon with Message.vi"("Already active? (F)"=w683, "Message"=w685, "Error In"=w680, "Target VI Refnum"=w684) -> ("Error Out"=w686:errorcluster)  [unwired: 7 in]
      n210 = Concatenate Strings(w670, " Hot Pixel Mask" ("string"), ".PNG" ("string")) -> (w696:string)
      n211 = Build Path(base path=w701, name or relative path=w696) -> (appended path=w700:path)
      n212 = call "Image File Dialog (Optional).vi"("Dialog?"=TRUE, "Error In"=w686, "Image File Format in"=Image_Save_File_Format."PNG", "Default file path in"=w700) -> ("Error Out"=w697:errorcluster, "Image File Format out"=w698:T25, "file path out"=w699:path)  [unwired: 5 in]
      n213 = call "AlliGator Save Hot Pixel Mask Image.vi"("error in (no error)"=w697, "Saved Image File Format"=w698, "File Path in"=w699, "Image Refnum in"=w672) -> ("Error Out"=w687:errorcluster, "File Path out"=w692:path)  [unwired: 6 in]
      n214 = call "Hide Animated Busy Icon with Message.vi"("Already active? (F)"=w683, "Error In"=w687, "Target VI reference"=w684) -> ("Error Out"=w666:errorcluster)  [unwired: 8 in]
      n215 = Format Into String(format string="Hot Pixel Mask Image saved to %s", error in=w666, w692) -> (resulting string=w688:string, error out=w693:errorcluster)  [unwired: 1 in]
    }
    frame "Image:Save Image Data as TIFF" {
      # "\"Save Image Data as TIFF\""
      n216 = in-place "In Place Element Structure" {
        in-place-border: [w735] -> w717
        in-place-border: [w734] -> w716
        in-place-border: [w733] -> w715
        in-place-border: [w732] -> w714
        in-place-border: [w731] -> w713
        n217 = in-place-dvr #6 ("Data Value Reference Read / Write Element")(w710) -> (w730:T30)  [unwired: 1 out]
        n218 = Unbundle By Name(w730) -> ("Type of Displayed Image"=w735:T36, "Gate Image Slide"=w731:u16, "Single Data Point Path"=w732:path, "Phasor Plot Image"=w733:T24, "Displayed Image"=w734:T24)
        n219 = in-place-dvr #6 ("Data Value Reference Read / Write Element")() -> (w709:refnum<data-value>)  [unwired: 1 in, 1 out]
      }
      n220 = call-poly "Variant to Data.vi"("Variant"=w726) -> ("Value"=w724:bool)  [unwired: 8 in]
      n221 = case shown="False" w724 {
        tunnel: w717 -> [w738 _]
        tunnel: [w737 AlliGator_Saved_TIFF_Image_Type."Phasor" ("Displayed Image")] -> w723
        tunnel: [w736 _] -> w720
        frame False {
          n222 = case shown="\"-\"" w738 {
            tunnel: [_ AlliGator_Saved_TIFF_Image_Type."Single Gate" ("Displayed Image") AlliGator_Saved_TIFF_Image_Type."Sum of All Gates" ("Displayed Image")] -> w737
            tunnel: [w739 _ _] -> w736
            frame "-" {
              n223 = xnode ("Error Ring")() -> ("error out"=w739:errorcluster)
            }
            frame "Single Gate", Default {
            }
            frame "Sum of All Gates" {
            }
          }
        }
        frame True {
        }
      }
      n224 = Select(t=w715, s=w724, f=w716) -> (s? t:f=w725:T24)
      n225 = call "Show Animated Busy Icon with Message.vi"("Already active? (F)"=w711, "Message"=w718, "Error In"=w720, "Target VI Refnum"=w719) -> ("Error Out"=w728:errorcluster)  [unwired: 7 in]
      n226 = call "AlliGator Save Image Data to File.vi"("Time Gate"=w713, "error in (no error)"=w728, "Saved TIFF Image"=w723, "Image"=w725, "File Path in"=w714) -> ("error out"=w721:errorcluster, "Output String"=w722:string, "Message"=w712:string)  [unwired: 3 in, 1 out]
      n227 = call "Hide Animated Busy Icon with Message.vi"("Already active? (F)"=w711, "Message"=w722, "Error In"=w721, "Target VI reference"=w719) -> ("Error Out"=w727:errorcluster)  [unwired: 7 in]
    }
    frame "Image:Save Image Overlay Only" {
      # "\"Save Image Overlay Only\""
      n228 = in-place "In Place Element Structure" {
        in-place-border: [w786] -> w759
        in-place-border: [w785] -> w758
        in-place-border: [w784] -> w757
        in-place-border: [w782] -> w749
        n229 = in-place-dvr #7 ("Data Value Reference Read / Write Element")(w750) -> (w783:T30, w782:errorcluster)
        n230 = Unbundle By Name(w783) -> ("Single Data Point Path"=w786:path, "[Time-Series Paths]"=w785:path[], "Current Dataset"=w784:i32)
        n231 = in-place-dvr #7 ("Data Value Reference Read / Write Element")() -> (w747:refnum<data-value>)  [unwired: 1 in, 1 out]
      }
      n232 = Unbundle By Name(w763) -> ("Registered Events Ctrl Refnums.Source Image Display"=w774:refnum<vi>)
      n233 = call-poly "Variant to Data.vi"("Variant"=w766) -> ("Value"=w765:bool)  [unwired: 8 in]
      n234 = property on="Property Node" class="ImageControl"(reference=w774, error in=w749) -> (reference out=w775:refnum<vi>, error out=w773:errorcluster, "Label.Text"=w780:string)
      n235 = call "AlliGator Get Destination Folder.vi"("Current Data Set (-1: single)"=w757, "Time-Series Paths"=w758, "Single Data Point Path"=w759) -> ("Data Point Name"=w777:string, "Destination Folder path"=w778:path)  [unwired: 6 in, 1 out]
      n236 = call "AlliGator Get Image File Format.vi"("Error In"=w773) -> ("error out"=w771:errorcluster, "File Extension (.xxx)"=w776:string, "Image File Format"=w772:T25)  [unwired: 7 in, 1 out]
      n237 = call "Show Animated Busy Icon with Message.vi"("Already active? (F)"=w751, "Message"=w753, "Error In"=w771, "Target VI Refnum"=w752) -> ("Error Out"=w754:errorcluster)  [unwired: 7 in]
      n238 = Concatenate Strings(w780, " Overlay " ("string"), w777, w776) -> (w764:string)
      n239 = Build Path(base path=w778, name or relative path=w764) -> (appended path=w770:path)
      n240 = call "Image File Dialog (Optional).vi"("Dialog?"=w765, "Error In"=w754, "Image File Format in"=w772, "Default file path in"=w770) -> ("Error Out"=w767:errorcluster, "Image File Format out"=w768:T25, "file path out"=w769:path)  [unwired: 5 in]
      n241 = call "Image Display Save Overlay.vi"("error in (no error)"=w767, "Saved Image File Format"=w768, "File Path in"=w769, "Display Image Control Refnum"=w775) -> ("Error Out"=w755:errorcluster, "File Path out"=w760:path)  [unwired: 6 in]
      n242 = call "Hide Animated Busy Icon with Message.vi"("Already active? (F)"=w751, "Error In"=w755, "Target VI reference"=w752) -> ("Error Out"=w748:errorcluster)  [unwired: 8 in]
      n243 = Format Into String(format string="Image overlay saved to %s", error in=w748, w760) -> (resulting string=w756:string, error out=w761:errorcluster)  [unwired: 1 in]
    }
    frame "Image:Save ROI" {
      # "\"Save ROI\""
      n244 = Unbundle By Name(w793) -> ("Dataset Control References.Current Data"=w792:refnum<vi>)
      n245 = Variant To Data(error in=w790, type=T27 {"Image Ctrl Ref"=refnum, "All ROIs?"=TRUE} ("Selected ROI"), Variant=w808) -> (data=w806:T27, error out=w789:errorcluster)
      n246 = Unbundle By Name(w806) -> ("Image Ctrl Ref"=w805:T28, "All ROIs?"=w803:bool)
      n247 = property on="Property Node" class="Str"(reference=w792, error in=w789) -> (error out=w788:errorcluster, "Value"=w791:string)  [unwired: 1 out]
      n248 = property on="Property Node" class="ImageControl"(reference=w805, error in=w788) -> (error out=w787:errorcluster, "Label.Text"=w804:string, "ROI"=w802:T67)  [unwired: 1 out]
      n249 = call "Show Animated Busy Icon with Message.vi"("Already active? (F)"=w794, "Message"=w797, "Error In"=w787, "Target VI Refnum"=w795) -> ("Error Out"=w798:errorcluster)  [unwired: 7 in]
      n250 = call "AlliGator Save ROI(s).vi"("Current Dataset Name"=w791, "Error In"=w798, "ROI Descriptor"=w802, "All ROIs?"=w803, "Image Label"=w804) -> ("Error Out"=w801:errorcluster, "Message"=w799:string)  [unwired: 5 in]
      n251 = call "Hide Animated Busy Icon with Message.vi"("Already active? (F)"=w794, "Error In"=w801, "Target VI reference"=w795) -> ("Error Out"=w796:errorcluster)  [unwired: 8 in]
    }
    frame "Image:Set Image Histogram Cursor Move Flag" {
      # "\"Image:Set Image Histogram Cursor Move Flag\""
      n252 = call-poly "Variant to Data.vi"("Variant"=w812) -> ("Value"=w811:bool)  [unwired: 8 in]
      n253 = call "AlliGator Image Contrast Status.vi"("Flag (in)"=w811, "Read/Write"=Read-Write."Write") -> ()  [unwired: 7 in, 1 out]
    }
    frame "Image:Set ROI Diameter" {
      # "\"Set ROI Diameter\""
      n254 = Unbundle By Name(w819) -> ("Registered Events Ctrl Refnums.Source Image Display"=w823:refnum<vi>)
      n255 = call "AlliGator Settings Storage.vi"("AlliGator Settings List"=AlliGator_Settings_List."Source Image:ROI Diameter") -> ("Error Out"=w822:errorcluster, "Variant Data out"=w826:variant)  [unwired: 9 in]
      n256 = call-poly "Variant to Data.vi"("Variant"=w826) -> ("Value"=w825:i32)  [unwired: 8 in]
      n257 = call "Image Display Set ROI Diameter.vi"("Error In"=w822, "ROI Diameter"=w825, "Display Image Control Refnum"=w823) -> ("Error Out"=w821:errorcluster)  [unwired: 8 in]
      n258 = Format Into String(format string=": %d", error in=w821, w825) -> (resulting string=w817:string, error out=w820:errorcluster)  [unwired: 1 in]
    }
    frame "Image:Set Source Image Mouse Move Flag" {
      # "\"Image:Set Source Image Mouse Move Flag\""
      n259 = call-poly "Variant to Data.vi"("Variant"=w832) -> ("Value"=w831:bool)  [unwired: 8 in]
      n260 = call "AlliGator Source Image Display Mouse Move Flag.vi"("Flag (in)"=w831, "Read/Write"=Read-Write."Write") -> ()  [unwired: 7 in, 1 out]
    }
    frame "Image:Show Phasor Calibration Map ROI Centers" {
      # "\"Image:Show Phasor Calibration Map ROI Centers\""
      n261 = Unbundle By Name(w839) -> ("Registered Events Ctrl Refnums.Source Image Display"=w838:refnum<vi>, "Dataset Control References.Source Image ROI Color"=w837:refnum<vi>)
      n262 = call "Show Animated Busy Icon with Message.vi"("Already active? (F)"=w845, "Message"=w844, "Target VI Refnum"=w846) -> ("Error Out"=w841:errorcluster)  [unwired: 8 in]
      n263 = call "AlliGator Show Phasor Calibration Map ROI Centers Overlay.vi"("Error In"=w841, "Source Image ROI Color"=w837, "Destination Image Control Refnum"=w838, "AlliGator IV DVR in"=w843) -> ("Error Out"=w840:errorcluster, "AlliGator IV DVR out"=w842:refnum<data-value>)  [unwired: 6 in]
      n264 = call "Hide Animated Busy Icon with Message.vi"("Already active? (F)"=w845, "Error In"=w840, "Target VI reference"=w846) -> ()  [unwired: 8 in, 1 out]
    }
    frame "Image:Source Image ROI Selection" {
      # "\"Source Image ROI Selection\""
      n265 = Variant To Data(Variant=w863) -> (data=w852:T77, error out=w862:errorcluster)  [unwired: 2 in]
      n266 = call "Show Animated Busy Icon with Message.vi"("Already active? (F)"=w858, "Error In"=w862, "Target VI Refnum"=w859) -> ("Error Out"=w860:errorcluster)  [unwired: 8 in]
      n267 = call "AlliGator Source Image Selection.vi"("AlliGator Ctrl Refnums"=w853, "error in (no error)"=w860, "ROI Selection Data"=w852) -> ("error out"=w851:errorcluster, "Alligator Queue Element out"=w856:T4[])  [unwired: 7 in]
      n268 = call "Hide Animated Busy Icon with Message.vi"("Already active? (F)"=w858, "Error In"=w851, "Target VI reference"=w859) -> ("Error Out"=w850:errorcluster)  [unwired: 8 in]
      n269 = call-poly "AlliGator Add Action(s) to Stack.vi"("Elements Order in Action Stack (Default: 2 BEFORE 1)"=Alligator_Elements_Order_in_Action_Stack."Enqueue 2 BEFORE 1", "Error In"=w850, "Alligator Queue Element 2"=w856, "Alligator Queue Element 1"=w857) -> ("Error Out"=w849:errorcluster, "Alligator Queue Element 1 (+ 2)"=w855:T4[])  [unwired: 6 in]
    }
    frame "Image:Source Image ROI Storage" {
      # "\"Source Image ROI Storage\""
      n270 = Variant To Data(type=AlliGator_ROI_Manager_Actions."Show All ROIs" ("Action"), Variant=w879) -> (data=w878:T21, error out=w871:errorcluster)  [unwired: 1 in]
      n271 = Unbundle By Name(w875) -> ("Registered Events Ctrl Refnums.Source Image Display"=w872:refnum<vi>)
      n272 = call "Image Display Get-Set ROI.vi"("Get(F)/Set"=FALSE ("Get(F)/Set(T)"), "Error In"=w871, "Image Display Refnum"=w872) -> ("Error Out"=w869:errorcluster, "ROI Descriptor out"=w866:T22, "Image Display Refnum (dup)"=w870:T28)  [unwired: 4 in, 2 out]
      n273 = call "ROI to Default ROI Name.vi"("Error In"=w869, "ROI"=w866) -> ("Error Out"=w881:errorcluster, "ROI Type String"=w880:string)  [unwired: 8 in]
      n274 = call-poly "AlliGator Source Image ROI Storage [PM].vi"("Error In"=w881, "Current ROI Descriptor"=w866, "Default Name (\"ROI\")"=w880, "Action"=w878) -> ("Error Out"=w876:errorcluster, "Current ROI Descriptor"=w874:T22, "Message"=w864:string)  [unwired: 1 in, 4 out]
      n275 = call "Image Display Get-Set ROI.vi"("Get(F)/Set"=TRUE ("Get(F)/Set(T)"), "Error In"=w876, "ROI Descriptor in"=w874, "Image Display Refnum"=w870) -> ("Error Out"=w873:errorcluster)  [unwired: 3 in, 4 out]
    }
    frame "Image:Store ROI" {
      # "\"Image:Merge All ROIs\""
      n276 = Bundle By Name(cluster=T4 {"AlliGator Q Event"=enum."Image:Source Image ROI Storage", "Data"=variant} ("Alligator Atomic Action"), "Data"=AlliGator_ROI_Manager_Actions."Store New ROI" ("Action")) -> (w887:T4)
      n277 = call-poly "AlliGator Add Action(s) to Stack.vi"("Elements Order in Action Stack (Default: 2 BEFORE 1)"=Alligator_Elements_Order_in_Action_Stack."Enqueue 2 BEFORE 1", "Error In"=w885, "Alligator Atomic Action"=w887, "Alligator Queue Element 1"=w893) -> ("Error Out"=w884:errorcluster, "Alligator Queue Element 1 (+ 2)"=w890:T4[])  [unwired: 6 in]
    }
    frame "Image:Update Image Profile Plots" {
      # "\"Update Image Profile Plots\""
      n278 = Unbundle By Name(w906) -> ("Registered Events Ctrl Refnums.Source Image Display"=w907:refnum<vi>, "Decay Fit Map Ctrl Refums.Decay Fit Parameter"=w905:refnum<vi>)
      n279 = property on="Property Node" class="Enum (strict)"(reference=w905, error in=w899) -> (error out=w900:errorcluster, "Value"=w904:T64)  [unwired: 1 out]
      n280 = call "Show Animated Busy Icon with Message.vi"("Already active? (F)"=w894, "Message"=w896, "Error In"=w900, "Target VI Refnum"=w895) -> ("Error Out"=w898:errorcluster)  [unwired: 7 in]
      n281 = call "AlliGator Send Plots to Image Profile Window.vi"("Image Control Refnum"=w907, "error in (no error)"=w898, "Fit Parameter"=w904, "AlliGator IV DVR in"=w903) -> ("error out"=w901:errorcluster, "AlliGator IV DVR out"=w902:refnum<data-value>)  [unwired: 6 in]
      n282 = call "Hide Animated Busy Icon with Message.vi"("Already active? (F)"=w894, "Error In"=w901, "Target VI reference"=w895) -> ("Error Out"=w897:errorcluster)  [unwired: 8 in]
    }
    frame "Image:Use ROI as Search Area" {
      # "\"Use ROI as Search Area\""
      n283 = Unbundle By Name(w911) -> ("Registered Events Ctrl Refnums.Source Image Display"=w912:refnum<vi>)
      n284 = call "AlliGator Store Search ROI.vi"("Display Image Control Refnum"=w912) -> ("Error Out"=w913:errorcluster, "Message"=w909:string)  [unwired: 8 in, 1 out]
    }
  }
  "AlliGator IV DVR out" <- w16
  "error out" <- w5
  "Script out" <- w9
  "Alligator Queue Elements" <- w8
  n285 = call "Message Style.vi"() -> ("Message Formatting"=w3:T2)
  n286 = call "AlliGator Package Notebook Messages.vi"("Message Formatting"=w3, "Message"=w2, "AlliGator Q Event in"="AlliGator Q Event in") -> ("[Notebook Message]"=→"[Notebook Message]":T1[])  [unwired: 8 in]
